vi "CRYGraph Property Window Octave.vi"(9 "TabName":string, 10 "Graph VI Ref":refnum<vi>) -> ()   [LabVIEW 2013]
uses:
  <vilib>/Utility/miscctls.llb/LVRowAndColumnTypeDef.ctl
panel:
  in  "SetFormat":bool
  in  "No Data":bool
  out "CursorLineStyle":string
  out "CursorLineWidth":string
  out "CursorPointStyle":string
  out "CursorStyle":string
  out "Scale Style":u8=5
  out "Interpolation":string
  out "PointStyle":string
  out "LineWidth":string
  out "LineStyle":string
  in  "Property Tab":T1(tab)
  in  "Background Color":u32(colorbox) caption="背景颜色"
  in  "Title Name":string caption="标题名字"
  in  "FormatAxis":u16(ring) items=["X-Axis", "Y-Axis"]
  in  "Notation":i32(listbox)
  in  "PrecisionType":u16(ring) items=["精度位数", "有效数字"]
  in  "PrecisionDigits":u16
  in  "Hide trailing zeros":bool caption="隐藏尾随零"
  in  "Exponent in multiples of 3":bool caption="指数"
  in  "Use minimum field width":bool caption="使用最小场宽度"
  in  "Field Width":u16
  in  "PadType":u16(ring) items=["在左加空格", "在右加空格", "在左加零"]
  in  "Ignore timestamp information":bool caption="忽略时间戳信息"
  in  "TimeFormat":u16(ring) items=["Custom time format", "System time format", "Time unused"]
  in  "Digits":u16 caption="a"
  in  "DateFormat":u16(ring) items=["Custom date format", "System date format", "Date unused"]
  in  "YMD":u16(slide)
  in  "YearShow":u16(slide)
  in  "AMFM":u16(slide)=1
  in  "HMS":u16(slide)=1
  in  "Point/Fill":u32(colorbox) caption="点/填充"
  in  "Fill to":i16(ring) caption="填写" items=["无"=-1, "零"=-2, "-无穷"=-3, "+无穷"=-4]
  in  "Items":u16(ring)
  out "Colors":bool caption="颜色"
  in  "Line":u32(colorbox) caption="线"
  in  "LineStyle4":bool
  in  "LineStyle3":bool
  in  "LineStyle2":bool
  in  "LineStyle0":bool
  in  "LineStyle1":bool
  in  "LineWidth5":bool
  in  "LineWidth1":bool
  in  "LineWidth4":bool
  in  "LineWidth3":bool
  in  "LineWidth2":bool
  in  "LineWidth0":bool
  in  "PointStyle16":bool
  in  "PointStyle15":bool
  in  "PointStyle14":bool
  in  "PointStyle13":bool
  in  "PointStyle12":bool
  in  "PointStyle11":bool
  in  "PointStyle10":bool
  in  "PointStyle9":bool
  in  "PointStyle8":bool
  in  "PointStyle7":bool
  in  "PointStyle6":bool
  in  "PointStyle5":bool
  in  "PointStyle4":bool
  in  "PointStyle3":bool
  in  "PointStyle2":bool
  in  "PointStyle1":bool
  in  "PointStyle0":bool
  in  "Interpolation4":bool
  in  "Interpolation5":bool
  in  "Interpolation3":bool
  in  "Interpolation2":bool
  in  "Interpolation1":bool
  in  "Interpolation0":bool
  in  "Show Plot":bool caption="显示绘图"
  in  "GridStyle":u16(ring)=4
  in  "Minor grid":u32(colorbox) caption="辅网格"
  in  "Major grid":u32(colorbox) caption="主网格"
  in  "Marker text":u32(colorbox) caption="标记文本"
  in  "Minor tick":u32(colorbox) caption="辅刻度"
  in  "Log":bool caption="对数"
  in  "Show scale":bool caption="显示缩放"
  in  "Show scale label":bool caption="显示缩放标签"
  in  "Maximum":dbl caption="最大值"
  in  "Minimum":dbl caption="最小值"
  in  "Autoscale":bool caption="自动缩放"
  in  "Axis Name":string caption="名字"
  in  "Axis":u16(ring)
  in  "Major tick":u32(colorbox) caption="主刻度"
  out "Grid Colors":bool caption="网格颜色"
  out "Scale Style and Colors":bool caption="缩放样式和颜色"
  in  "Show Cursors":bool caption="显示游标"
  in  "Cursor Tab":enum32{"Page 1"}(tab)
  in  "CursorPointStyle16":bool
  in  "CursorPointStyle15":bool
  in  "CursorPointStyle14":bool
  in  "CursorPointStyle13":bool
  in  "CursorPointStyle12":bool
  in  "CursorPointStyle11":bool
  in  "CursorPointStyle10":bool
  in  "CursorPointStyle9":bool
  in  "CursorPointStyle8":bool
  in  "CursorPointStyle7":bool
  in  "CursorPointStyle6":bool
  in  "CursorPointStyle5":bool
  in  "CursorPointStyle4":bool
  in  "CursorPointStyle3":bool
  in  "CursorPointStyle2":bool
  in  "CursorPointStyle1":bool
  in  "CursorPointStyle0":bool
  in  "CursorLineWidth5":bool
  in  "CursorLineWidth1":bool
  in  "CursorLineWidth4":bool
  in  "CursorLineWidth3":bool
  in  "CursorLineWidth2":bool
  in  "CursorLineWidth0":bool
  in  "CursorLineStyle4":bool
  in  "CursorLineStyle3":bool
  in  "CursorLineStyle2":bool
  in  "CursorLineStyle0":bool
  in  "CursorLineStyle1":bool
  in  "Cursor Items":u16(ring)
  in  "CursorStyle8":bool
  in  "CursorStyle4":bool
  in  "CursorStyle5":bool
  in  "CursorStyle7":bool
  in  "CursorStyle6":bool
  in  "CursorStyle3":bool
  in  "CursorStyle2":bool
  in  "CursorStyle1":bool
  in  "CursorStyle0":bool
  in  "Cursor color":u32(colorbox) caption="游标颜色"
  in  "Linked to plot:":u16(ring) caption="连接到游标"
  in  "Link Cursors":bool
  in  "OK":bool
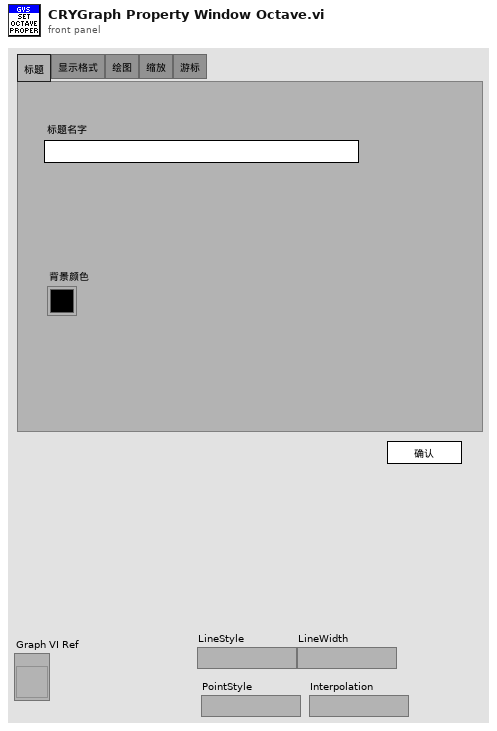
[diagram p1: front panel]
types:
  T1 = enum32{"Title", "Format and Precision", "Plot", "Scale", "Cursor"}
  T2 = enum32{"Page Enabled", "Page Disabled", "Page Disabled & Grayed"}
  T3 = enum8{"Enabled", "Disabled", "Disabled and Grayed Out"}
  T4 = typedef "LVRowAndColumnTypeDef.ctl" = cluster{"Row":i32, "Column":i32}
  T5 = typedef "CRYData Cluster.ctl" = cluster{"Name":string, "Curve":cluster{"x":dbl, "y":dbl, "z":dbl}[], "X data":u16, "Y data":u16, "Z data":u16, "X axis":u16, "Y axis":u16, "Z axis":u16, "X unit":string, "Y unit":string, "Z unit":string, "X dB ref":dbl, "Y dB ref":dbl, "Z dB ref":dbl, "single val":bool, "protected":bool, "display X":bool, "display Y":bool, "display Z":bool, "Test Info":string, "Step No.":i32, "Plot Settings":cluster{"Color":u32, "Interpolation":u8, "Point Style":u8, "Line Style":u8, "Point Color":u32, "Line Width":u8, "Bar Plot Style":u8, "Fill To":i16}, "AutoProtect":bool}
  T6 = cluster{"Notation":i32, "PrecisionType":u16, "PrecisionDigits":u16, "Hide trailing zeros":bool, "Exponent in multiples of 3":bool, "Field Width":u16, "PadType":u16, "Use minimum field width":bool, "TimeFormat":u16, "AMFM":u16, "HMS":u16, "Digits":u16, "DateFormat":u16, "YMD":u16, "YearShow":u16}
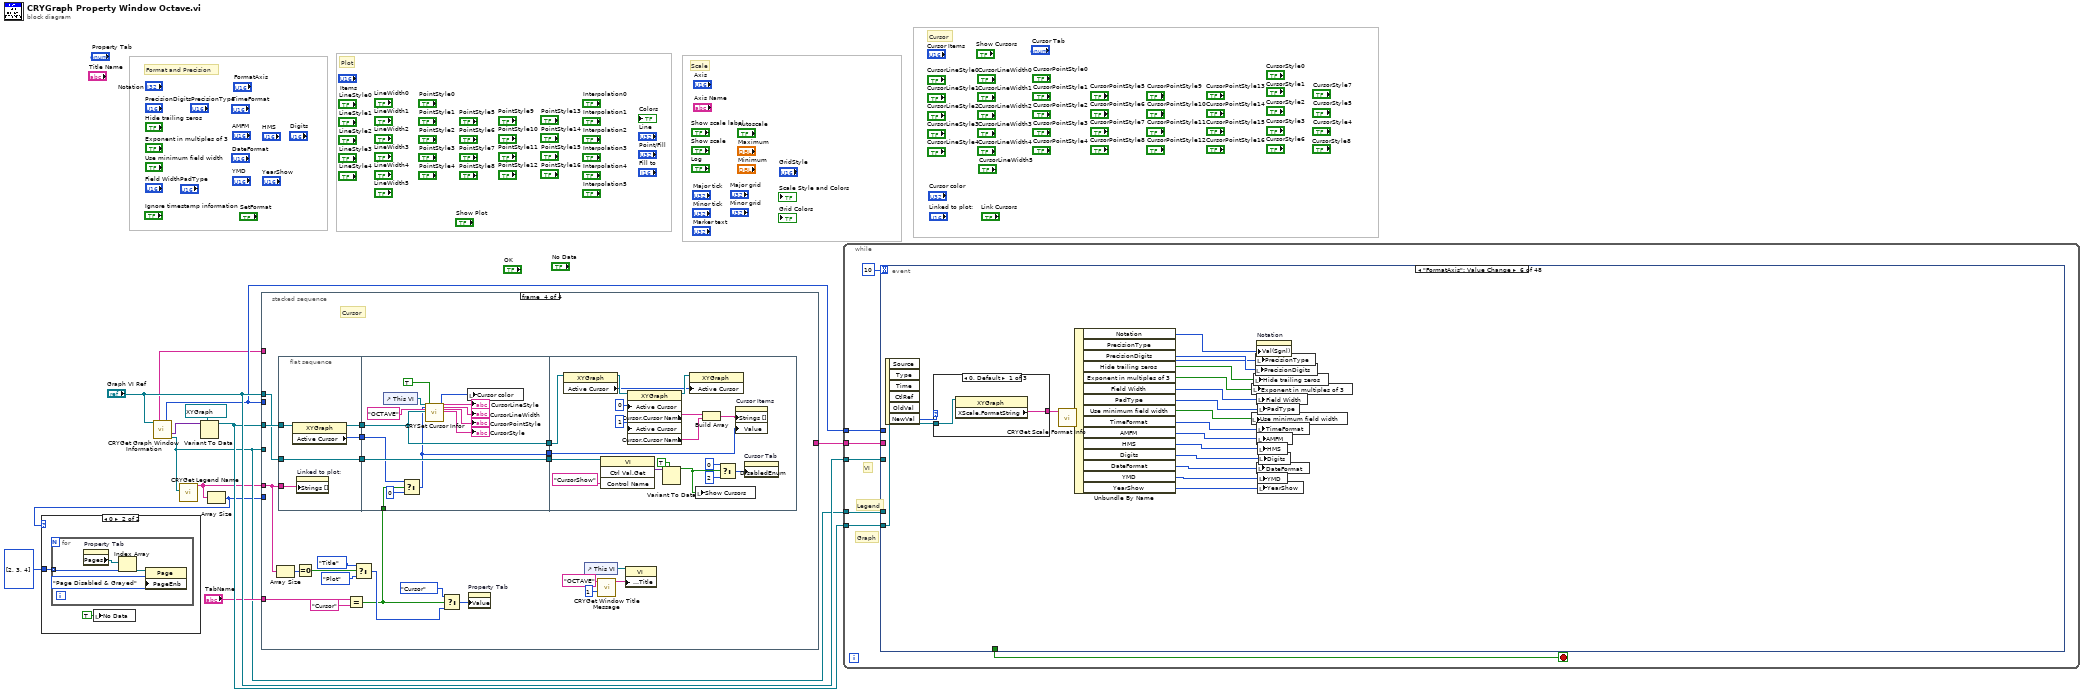
[diagram p0: block diagram]
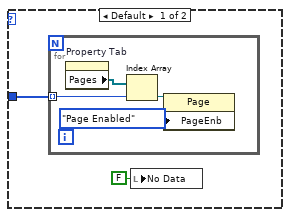
[diagram p2: hidden frame]
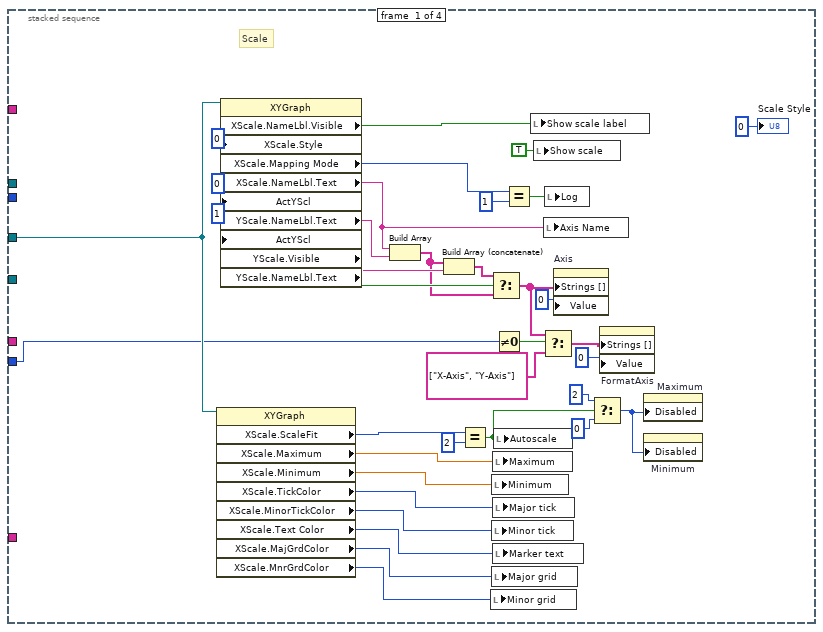
[diagram p3: hidden frame]
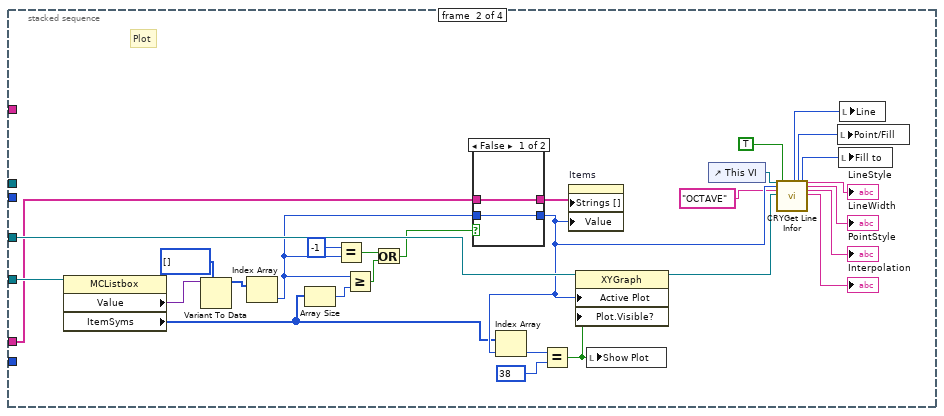
[diagram p4: hidden frame]
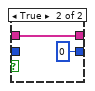
[diagram p5: hidden frame]
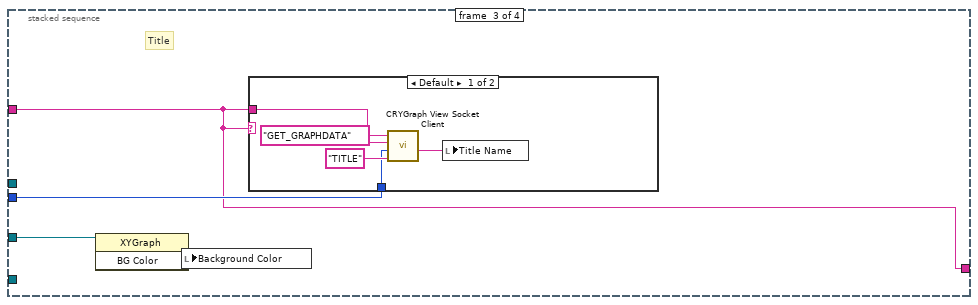
[diagram p6: hidden frame]
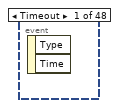
[diagram p8: hidden frame]
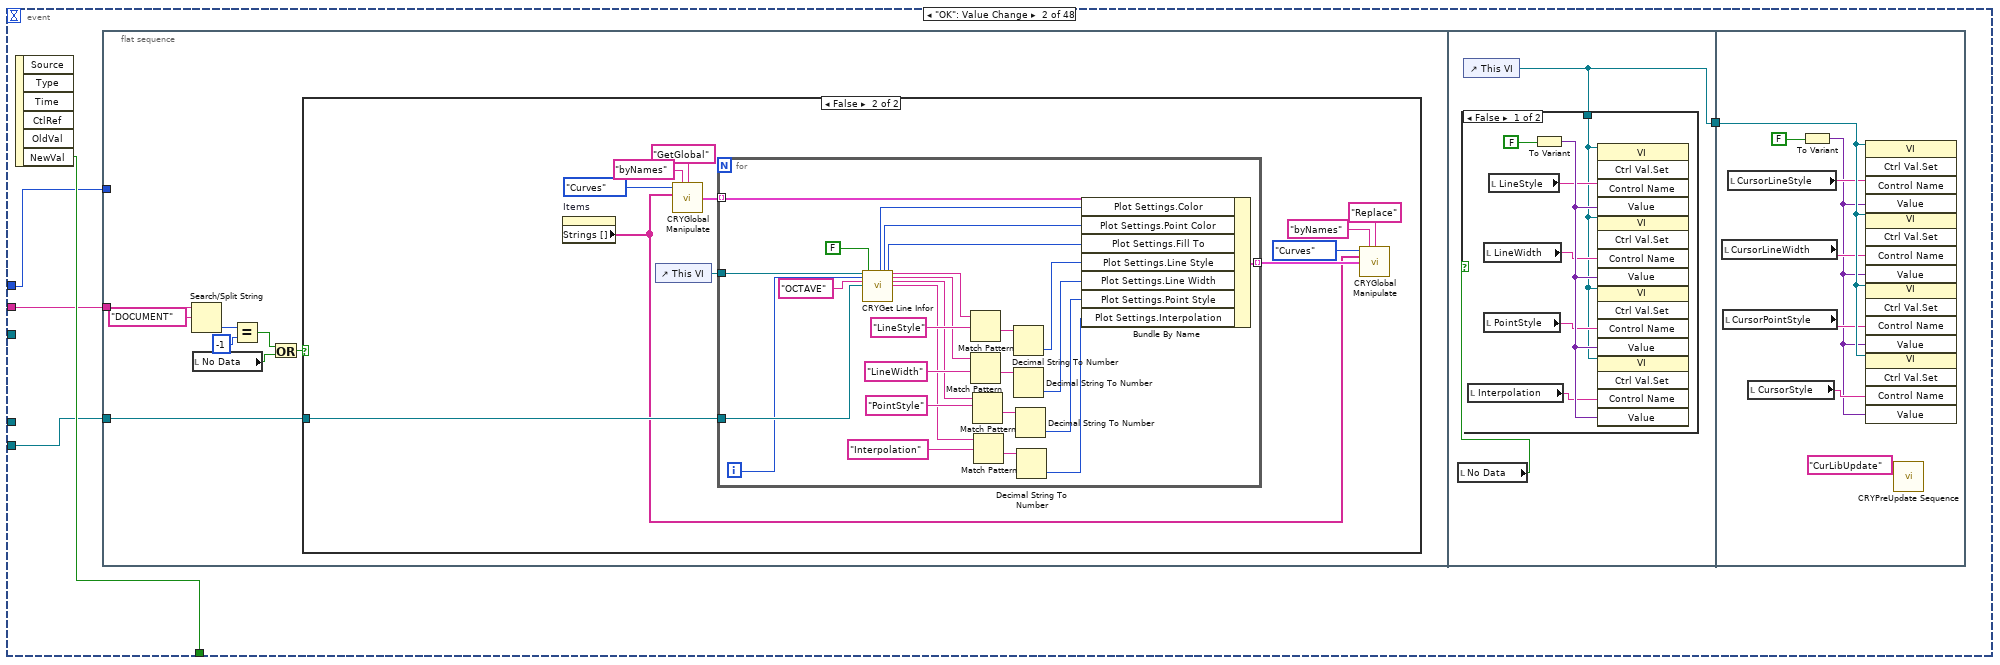
[diagram p9: hidden frame]
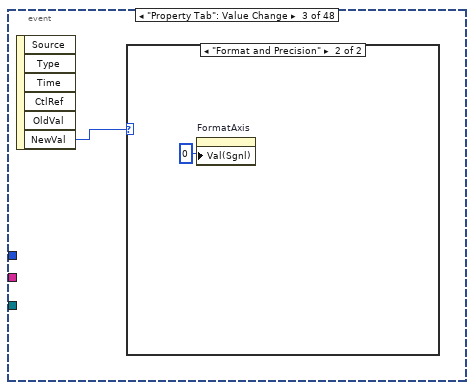
[diagram p12: hidden frame]
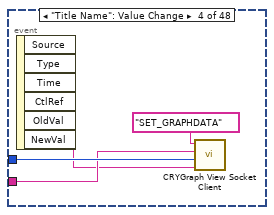
[diagram p14: hidden frame]
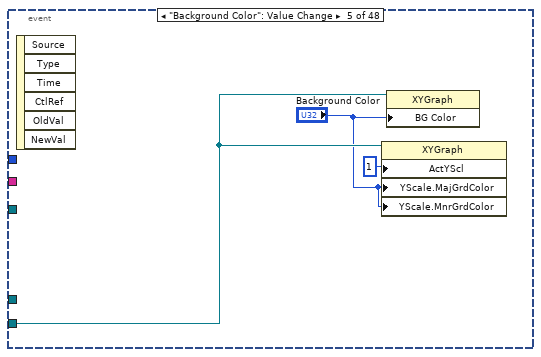
[diagram p15: hidden frame]
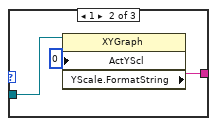
[diagram p16: hidden frame]
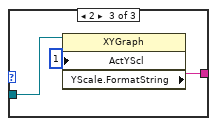
[diagram p17: hidden frame]
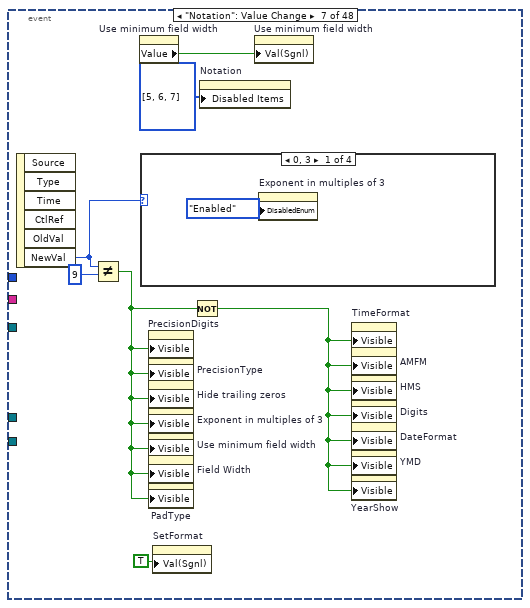
[diagram p18: hidden frame]
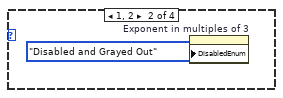
[diagram p19: hidden frame]
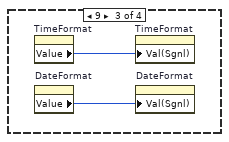
[diagram p20: hidden frame]
diagram:
  # "Format and Precision"
  # "Cursor"
  # "Scale"
  # "Plot"
  n1 = call "CRYGet Graph Window Information.vi"("pGraph VI In"="Graph VI Ref") -> ("Queue Name Out"=w9:string, "Graph Number Out"=w10:i32, "Graph Control Ref Out"=w2:variant, "Legend Ref Out"=w6:refnum<vi>)  [unwired: 2 in, 9 out]
  n2 = call "CRYGet Legend Name.vi"("MCListbox Refnum"=w6) -> ("Names Out"=w5:string[])  [unwired: 1 in, 9 out]
  n3 = Variant To Data(type=refnum<vi> refnum ("XY Graph"), Variant=w2) -> (data=w11:refnum<vi>)  [unwired: 1 in, 1 out]
  n4 = Array Size(array=w5) -> (size(s)=w4:i32)
  n5 = case shown="0" w4 {
    tunnel: i32[] [2, 3, 4] -> [w13 w19]
    frame Default {
      n6 = for {
        tunnel: w13 -> [w16] mode=indexing
        n7 = property on="Property Tab" class="TabCtl (strict)"() -> ("Pages"=w15:refnum<vi>[])  [unwired: 2 in, 2 out]
        n8 = Index Array(array=w15, index=w16) -> (element=w17:refnum<vi>)
        n9 = property class="Page"(reference=w17, "PageEnb"=T2."Page Enabled" ("Page Enabled State")) -> ()  [unwired: 1 in, 2 out]
      }
      n10 = local write "No Data"(FALSE ("No Data")) -> ()
    }
    frame 0 {
      n11 = for {
        tunnel: w19 -> [w21] mode=indexing
        n12 = property on="Property Tab" class="TabCtl (strict)"() -> ("Pages"=w22:refnum<vi>[])  [unwired: 2 in, 2 out]
        n13 = Index Array(array=w22, index=w21) -> (element=w23:refnum<vi>)
        n14 = property class="Page"(reference=w23, "PageEnb"=T2."Page Disabled & Grayed" ("Page Enabled State")) -> ()  [unwired: 1 in, 2 out]
      }
      n15 = local write "No Data"(TRUE ("No Data")) -> ()
    }
  }
  n16 = stacked-sequence {
    tunnel: w11 -> [w60 w88 w97 w125]
    tunnel: "Graph VI Ref" -> [_ _ _ w122]
    tunnel: w6 -> [_ w89 _ _]
    tunnel: w10 -> [_ _ w95 _]
    tunnel: w9 -> [_ _ w94 _]
    tunnel: [_ _ w94 _] -> w8
    tunnel: "TabName" -> [_ _ _ w120]
    tunnel: w5 -> [_ w87 _ w114]
    tunnel: w4 -> [w29 _ _ _]
    frame #0 {
      # "Scale"
      n17 = property class="XYGraph"(reference=w60) -> ("XScale.ScaleFit"=w47:u8, "XScale.Maximum"=w46:dbl, "XScale.Minimum"=w45:dbl, "XScale.TickColor"=w44:u32, "XScale.MinorTickColor"=w43:u32, "XScale.Text Color"=w42:u32, "XScale.MajGrdColor"=w41:u32, "XScale.MnrGrdColor"=w40:u32)  [unwired: 1 in, 2 out]
      n18 = property class="XYGraph"(reference=w60, "XScale.Style"=u8 0 ("X Scale.Style"), "ActYScl"=0 ("Active Y Scale"), "ActYScl"=1 ("Active Y Scale")) -> ("XScale.NameLbl.Visible"=w58:bool, "XScale.Mapping Mode"=w56:u8, "XScale.NameLbl.Text"=w53:string, "YScale.NameLbl.Text"=w51:string, "YScale.Visible"=w34:bool, "YScale.NameLbl.Text"=w33:string)  [unwired: 1 in, 2 out]
      n19 = Build Array(w53, w51) -> (w31:string[])
      n20 = Build Array (concatenate)(w31, w33) -> (w32:string[])
      n21 = Equal?(x=w47, y=u8 2 ("X Scale.Scale Fit")) -> (x = y?=w36:bool)
      n22 = Select(t=w32, s=w34, f=w31) -> (s? t:f=w27:string[])
      n23 = local write "Minor grid"(w40) -> ()
      n24 = local write "Minimum"(w45) -> ()
      n25 = local write "Minor tick"(w43) -> ()
      n26 = local write "Major grid"(w41) -> ()
      n27 = local write "Maximum"(w46) -> ()
      n28 = local write "Major tick"(w44) -> ()
      n29 = local write "Marker text"(w42) -> ()
      n30 = Not Equal To 0?(x=w29) -> (x != 0?=w28:bool)
      n31 = local write "Autoscale"(w36) -> ()
      n32 = Equal?(x=w56, y=u8 1) -> (x = y?=w57:bool)
      n33 = local write "Show scale label"(w58) -> ()
      n34 = local write "Show scale"(TRUE ("Show scale")) -> ()
      n35 = Select(t=w27, s=w28, f=string[] ["X-Axis", "Y-Axis"]) -> (s? t:f=w25:string[])
      n36 = local write "Axis Name"(w53) -> ()
      n37 = local write "Log"(w57) -> ()
      n38 = property on="Axis" class="Ring (strict)"("Strings []"=w27, "Value"=0) -> ()  [unwired: 2 in, 2 out]
      n39 = Select(t=u8 2 ("X Scale.Scale Fit"), s=w36, f=u8 0 ("X Scale.Scale Fit")) -> (s? t:f=w37:u8)
      n40 = property on="FormatAxis" class="Ring (strict)"("Strings []"=w25, "Value"=0) -> ()  [unwired: 2 in, 2 out]
      n41 = property on="Maximum" class="DigNum (strict)"("Disabled"=w37) -> ()  [unwired: 2 in, 2 out]
      n42 = property on="Minimum" class="DigNum (strict)"("Disabled"=w37) -> ()  [unwired: 2 in, 2 out]
      "Scale Style" <- u8 0 ("X Scale.Scale Fit")
    }
    frame #1 {
      # "Plot"
      n43 = property class="MCListbox"(reference=w89) -> ("Value"=w81:variant, "ItemSyms"=w63:i32[])  [unwired: 1 in, 2 out]
      n44 = Variant To Data(type=i32[] [], Variant=w81) -> (data=w68:i32[])  [unwired: 1 in, 1 out]
      n45 = Index Array(array=w68) -> (element=w61:i32)  [unwired: 1 in]
      n46 = Array Size(array=w63) -> (size(s)=w66:i32)
      n47 = Equal?(x=-1, y=w61) -> (x = y?=w65:bool)
      n48 = Greater Or Equal?(x=w61, y=w66) -> (x >= y?=w64:bool)
      n49 = Or(x=w65, y=w64) -> (x .or. y?=w62:bool)
      n50 = case shown="False" w62 {
        tunnel: w87 -> [w91 w93]
        tunnel: [w91 w93] -> w86
        tunnel: [w90 0 ("Value")] -> w80
        tunnel: w61 -> [w90 _]
        frame False {
        }
        frame True {
        }
      }
      n51 = Index Array(array=w63, index=w80) -> (element=w83:i32)
      n52 = Equal?(x=w83, y=38) -> (x = y?=w82:bool)
      n53 = property on="Items" class="Ring (strict)"("Strings []"=w86, "Value"=w80) -> ()  [unwired: 2 in, 2 out]
      n54 = property class="XYGraph"(reference=w88, "Active Plot"=w80, "Plot.Visible?"=w82) -> (reference out=w85:refnum<vi>)  [unwired: 1 in, 1 out]
      n55 = local write "Show Plot"(w82) -> ()
      n56 = control-ref of="This VI"() -> (w79:refnum<vi>)
      n57 = call "CRYGet Line Infor.vi"("This VI"=w79, "Active Plot Number"=w80, "Graph Type"="OCTAVE", "XY Graph Control Ref"=w85, "Property Set?"=TRUE) -> ("Line"=w72:u32, "Point/Fill"=w70:u32, "Fill to"=w71:i16, "LineStyle"=→"LineStyle":string, "LineWidth"=→"LineWidth":string, "PointStyle"=→"PointStyle":string, "Interpolation"=→"Interpolation":string)  [unwired: 16 in]
      n58 = local write "Point/Fill"(w70) -> ()
      n59 = local write "Fill to"(w71) -> ()
      n60 = local write "Line"(w72) -> ()
    }
    frame #2 {
      # "Title"
      n61 = property class="XYGraph"(reference=w97) -> ("BG Color"=w96:u32)  [unwired: 1 in, 2 out]
      n62 = local write "Background Color"(w96) -> ()
      n63 = case shown="Default" w94 {
        tunnel: w95 -> [w100 _]
        tunnel: w94 -> [w99 _]
        frame Default {
          n64 = call "CRYGraph View Socket Client.vi"("sOption"="TITLE", "nData"=w100, "sData"=w99, "sAction"="GET_GRAPHDATA") -> ("sData Out"=w98:string)  [unwired: 4 in, 3 out]
          n65 = local write "Title Name"(w98) -> ()
        }
        frame "test DataView" {
        }
      }
    }
    frame #3 {
      # "Cursor"
      n66 = Array Size(array=w114) -> (size(s)=w121:i32)
      n67 = flat-sequence {
        tunnel: w122 -> [w130]
        tunnel: w125 -> [w128]
        tunnel: [w127] -> w116
        tunnel: [w130] -> w115
        tunnel: w114 -> [w129]
        tunnel: [w126] -> w112
        tunnel: [w144] -> w124
        tunnel: [w135] -> w123
        tunnel: w116 -> [w144]
        tunnel: w115 -> [w135]
        tunnel: w113 -> [w133]
        tunnel: w112 -> [w132]
        tunnel: [w131] -> w111
        tunnel: w124 -> [w148]
        tunnel: w123 -> [w154]
        tunnel: w111 -> [w145]
        frame #0 {
          n68 = property class="XYGraph"(reference=w128) -> (reference out=w127:refnum<vi>, "Active Cursor"=w126:u32)  [unwired: 1 in, 1 out]
          n69 = property on="Linked to plot:" class="Ring (strict)"("Strings []"=w129) -> ()  [unwired: 2 in, 2 out]
        }
        frame #1 {
          n70 = control-ref of="This VI"() -> (w143:refnum<vi>)
          n71 = Select(t=w132, s=w133, f=u32 0 ("Active Cursor")) -> (s? t:f=w131:u32)
          n72 = call "CRYSet Cursor Infor.vi"("This VI"=w143, "Active Cursor"=w131, "Graph Type"="OCTAVE", "XY Graph Ref"=w144, "Property Set?"=TRUE) -> ("Cursor Color"=w136:u32, "CursorLineStyle"=→"CursorLineStyle":string, "CursorLineWidth"=→"CursorLineWidth":string, "CursorPointStyle"=→"CursorPointStyle":string, "CursorStyle"=→"CursorStyle":string)  [unwired: 17 in, 1 out]
          n73 = local write "Cursor color"(w136) -> ()
        }
        frame #2 {
          n74 = property class="XYGraph"(reference=w148) -> (reference out=w147:refnum<vi>, "Active Cursor"=w146:u32)  [unwired: 1 in, 1 out]
          n75 = invoke class="VI" method="Ctrl Val.Get"(reference=w154, "Control Name"="CursorShow") -> ("Get Control Value Variant"=w152:variant)  [unwired: 2 in, 3 out]
          n76 = property class="XYGraph"(reference=w147, "Active Cursor"=u32 0, "Active Cursor"=u32 1) -> (reference out=w149:refnum<vi>, "Cursor.Cursor Name"=w157:string, "Cursor.Cursor Name"=w158:string)  [unwired: 1 in, 1 out]
          n77 = Variant To Data(type=TRUE ("Visible"), Variant=w152) -> (data=w150:bool)  [unwired: 1 in, 1 out]
          n78 = property class="XYGraph"(reference=w149, "Active Cursor"=w146) -> ()  [unwired: 1 in, 2 out]
          n79 = local write "Show Cursors"(w150) -> ()
          n80 = Build Array(w157, w158) -> (w159:string[])
          n81 = Select(t=0, s=w150, f=2) -> (s? t:f=w160:i32)
          n82 = property on="Cursor Items" class="Ring (strict)"("Strings []"=w159, "Value"=w145) -> ()  [unwired: 2 in, 2 out]
          n83 = property on="Cursor Tab" class="TabCtl (strict)"("DisabledEnum"=w160) -> ()  [unwired: 2 in, 2 out]
        }
      }
      n84 = Equal To 0?(x=w121) -> (x = 0?=w118:bool)
      n85 = Equal?(x=w120, y="Cursor" ("Graph Type")) -> (x = y?=w113:bool)
      n86 = Select(t=T1."Title" ("Tab Control"), s=w118, f=T1."Plot" ("Tab Control")) -> (s? t:f=w117:T1)
      n87 = Select(t=T1."Cursor" ("Tab Control"), s=w113, f=w117) -> (s? t:f=w110:T1)
      n88 = property on="Property Tab" class="TabCtl (strict)"("Value"=w110) -> ()  [unwired: 2 in, 2 out]
      n89 = control-ref of="This VI"() -> (w103:refnum<vi>)
      n90 = call "CRYGet Window Title Message.vi"("No"=1 ("Error No"), "Kind"="OCTAVE") -> ("Multibyte String"=w104:string)  [unwired: 4 in, 5 out]
      n91 = property class="VI"(reference=w103, "Front Panel.Title"=w104) -> ()  [unwired: 1 in, 2 out]
    }
  }
  n92 = while {
    tunnel: w11 -> [w168]
    tunnel: "Graph VI Ref" -> [w167]
    tunnel: w6 -> [w165]
    tunnel: w8 -> [w164]
    tunnel: w10 -> [w163]
    stop <- w169 stop-if-true
    # "VI"
    # "Legend"
    # "Graph"
    n93 = event shown="[5] \"FormatAxis\": Value Change" {
      selector: _ -> [_ _ _ _ _ _ _ _ _ _ _ _ _ _ _ _ _ _ _ _ _ _ _ _ _ _ _ _ _ _ _ _ _ _ _ _ _ _ _ _ _ _ _ _ _ _ _ _]
      dyn-events: _ -> [_ _ _ _ _ _ _ _ _ _ _ _ _ _ _ _ _ _ _ _ _ _ _ _ _ _ _ _ _ _ _ _ _ _ _ _ _ _ _ _ _ _ _ _ _ _ _ _]
      timeout: 10 -> [_ _ _ _ _ _ _ _ _ _ _ _ _ _ _ _ _ _ _ _ _ _ _ _ _ _ _ _ _ _ _ _ _ _ _ _ _ _ _ _ _ _ _ _ _ _ _ _]
      tunnel: [_ w174 _ _ _ _ _ _ _ _ _ _ _ _ _ _ _ _ _ _ _ _ _ _ _ _ _ _ _ _ _ _ _ _ _ _ _ _ _ _ _ _ _ _ _ _ _ _] -> w169
      tunnel: w168 -> [_ w173 _ _ w244 w255 _ _ _ _ _ _ _ _ _ w330 w476 w508 w540 w572 w602 w639 w649 w659 w676 w698 w742 w754 w769 w781 w795 w807 w818 w829 w839 w851 w869 w906 w917 _ w934 w954 w975 w996 w1017 w1042 w1051 _]
      tunnel: w167 -> [_ _ _ _ _ _ _ _ _ _ _ _ _ _ _ _ _ _ _ _ _ _ _ _ _ _ _ _ _ _ _ _ _ _ _ _ w863 _ _ w930 _ _ _ _ _ w1043 _ _]
      tunnel: w165 -> [_ _ _ _ _ _ _ _ _ _ _ _ _ _ _ _ w475 w507 w539 w571 w604 w638 w645 w657 w673 _ _ _ _ _ _ _ _ _ _ _ _ _ _ _ _ _ _ _ _ _ _ _]
      tunnel: w164 -> [_ w171 _ w240 _ _ _ _ _ _ _ _ _ _ _ _ w474 w506 w538 w570 _ w632 w647 w656 _ _ _ _ _ _ _ _ _ _ _ _ _ _ _ _ _ _ _ _ _ _ _ _]
      tunnel: w163 -> [_ w170 _ w241 _ _ _ _ _ _ _ _ _ _ _ _ _ _ _ _ _ _ _ _ _ _ _ _ _ _ _ _ _ _ _ _ _ _ _ _ _ _ _ _ _ _ _ _]
      event Timeout {
        n94 = event-data() -> ()  [unwired: 3 out]
      }
      event "OK": Value Change {
        n95 = event-data() -> ("NewVal"=w174:bool)  [unwired: 6 out]
        n96 = flat-sequence {
          tunnel: w173 -> [w175]
          tunnel: w171 -> [w177]
          tunnel: w170 -> [_]
          tunnel: [w221] -> w172
          tunnel: w172 -> [w236]
          frame #0 {
            n97 = Search/Split String(string=w177, search string/char (-)="DOCUMENT" ("regular expression")) -> (offset of match=w181:i32)  [unwired: 1 in, 2 out]
            n98 = local read "No Data"() -> (w178:bool)
            n99 = Equal?(x=w181, y=-1) -> (x = y?=w179:bool)
            n100 = Or(x=w179, y=w178) -> (x .or. y?=w176:bool)
            n101 = case shown="False" w176 {
              tunnel: w175 -> [_ w192]
              frame True {
              }
              frame False {
                n102 = property on="Items" class="Ring (strict)"() -> ("Strings []"=w184:string[])  [unwired: 2 in, 2 out]
                n103 = control-ref of="This VI"() -> (w193:refnum<vi>)
                n104 = call "CRYGlobal Manipulate.vi"("Type"=enum16{"Curves", "Values", "Results", "WFM"}."Curves", "sOption"="byNames", "sAction"="GetGlobal", "sData"=w184) -> ("Curves Out"=w188:T5[])  [unwired: 5 in, 6 out]
                n105 = for {
                  tunnel: w193 -> [w218]
                  tunnel: w192 -> [w217]
                  tunnel: w188 -> [w195] mode=indexing
                  tunnel: [w194] -> w187 mode=indexing
                  i -> [w201]
                  n106 = call "CRYGet Line Infor.vi"("This VI"=w218, "Active Plot Number"=w201, "Graph Type"="OCTAVE", "XY Graph Control Ref"=w217, "Property Set?"=FALSE) -> ("Line"=w196:u32, "Point/Fill"=w197:u32, "Fill to"=w198:i16, "LineStyle"=w208:string, "LineWidth"=w204:string, "PointStyle"=w203:string, "Interpolation"=w202:string)  [unwired: 16 in]
                  n107 = Match Pattern(string=w208, regular expression="LineStyle") -> (after substring=w214:string)  [unwired: 4 out]
                  n108 = Match Pattern(string=w204, regular expression="LineWidth") -> (after substring=w215:string)  [unwired: 4 out]
                  n109 = Match Pattern(string=w203, regular expression="PointStyle") -> (after substring=w213:string)  [unwired: 4 out]
                  n110 = Match Pattern(string=w202, regular expression="Interpolation") -> (after substring=w210:string)  [unwired: 4 out]
                  n111 = Decimal String To Number(string=w214) -> (number=w207:i32)  [unwired: 3 out]
                  n112 = Decimal String To Number(string=w215) -> (number=w206:i32)  [unwired: 3 out]
                  n113 = Decimal String To Number(string=w213) -> (number=w205:i32)  [unwired: 3 out]
                  n114 = Decimal String To Number(string=w210) -> (number=w200:i32)  [unwired: 3 out]
                  n115 = Bundle By Name(cluster=w195, "Plot Settings.Color"=w196, "Plot Settings.Point Color"=w197, "Plot Settings.Fill To"=w198, "Plot Settings.Line Style"=w207, "Plot Settings.Line Width"=w206, "Plot Settings.Point Style"=w205, "Plot Settings.Interpolation"=w200) -> (w194:T5)
                }
                n116 = call "CRYGlobal Manipulate.vi"("Type"=enum16{"Curves", "Values", "Results", "WFM"}."Curves", "sOption"="byNames", "sAction"="Replace", "sData"=w184, "Curves"=w187) -> ()  [unwired: 4 in, 7 out]
              }
            }
          }
          frame #1 {
            n117 = local read "No Data"() -> (w220:bool)
            n118 = control-ref of="This VI"() -> (w221:refnum<vi>)
            n119 = case shown="False" w220 {
              tunnel: w221 -> [w222 _]
              frame False {
                n120 = local read "Interpolation"() -> (w223:string)
                n121 = local read "LineWidth"() -> (w225:string)
                n122 = local read "PointStyle"() -> (w224:string)
                n123 = local read "LineStyle"() -> (w226:string)
                n124 = To Variant(anything=FALSE) -> (Variant=w228:variant)
                n125 = invoke class="VI" method="Ctrl Val.Set"(reference=w222, "Control Name"=w226, "Value"=w228) -> ()  [unwired: 2 in, 5 out]
                n126 = invoke class="VI" method="Ctrl Val.Set"(reference=w222, "Control Name"=w225, "Value"=w228) -> ()  [unwired: 2 in, 5 out]
                n127 = invoke class="VI" method="Ctrl Val.Set"(reference=w222, "Control Name"=w224, "Value"=w228) -> ()  [unwired: 2 in, 5 out]
                n128 = invoke class="VI" method="Ctrl Val.Set"(reference=w222, "Control Name"=w223, "Value"=w228) -> ()  [unwired: 2 in, 5 out]
              }
              frame True {
              }
            }
          }
          frame #2 {
            n129 = local read "CursorLineWidth"() -> (w233:string)
            n130 = local read "CursorPointStyle"() -> (w234:string)
            n131 = local read "CursorLineStyle"() -> (w232:string)
            n132 = local read "CursorStyle"() -> (w235:string)
            n133 = To Variant(anything=FALSE) -> (Variant=w230:variant)
            n134 = invoke class="VI" method="Ctrl Val.Set"(reference=w236, "Control Name"=w232, "Value"=w230) -> ()  [unwired: 2 in, 5 out]
            n135 = invoke class="VI" method="Ctrl Val.Set"(reference=w236, "Control Name"=w233, "Value"=w230) -> ()  [unwired: 2 in, 5 out]
            n136 = invoke class="VI" method="Ctrl Val.Set"(reference=w236, "Control Name"=w234, "Value"=w230) -> ()  [unwired: 2 in, 5 out]
            n137 = invoke class="VI" method="Ctrl Val.Set"(reference=w236, "Control Name"=w235, "Value"=w230) -> ()  [unwired: 2 in, 5 out]
            n138 = call "CRYPreUpdate Sequence.vi"("EventName"="CurLibUpdate") -> ()  [unwired: 15 in]
          }
        }
      }
      event "Property Tab": Value Change {
        n139 = event-data() -> ("NewVal"=w237:T1)  [unwired: 6 out]
        n140 = case shown="\"Format and Precision\"" w237 {
          frame "Title", Default {
          }
          frame "Format and Precision" {
            n141 = property on="FormatAxis" class="Ring (strict)"("Val(Sgnl)"=u16 0 ("Value (Signaling)")) -> ()  [unwired: 2 in, 2 out]
          }
        }
      }
      event "Title Name": Value Change {
        n142 = event-data() -> ("NewVal"=w239:string)  [unwired: 6 out]
        n143 = call "CRYGraph View Socket Client.vi"("sOption"=w239, "nData"=w241, "sData"=w240, "sAction"="SET_GRAPHDATA") -> ()  [unwired: 4 in, 4 out]
      }
      event "Background Color": Value Change {
        n144 = event-data() -> ()  [unwired: 7 out]
        n145 = property on="Property Node" class="XYGraph"(reference=w244, "ActYScl"=1 ("Active Y Scale"), "YScale.MajGrdColor"="Background Color", "YScale.MnrGrdColor"="Background Color") -> ()  [unwired: 1 in, 2 out]
        n146 = property class="XYGraph"(reference=w244, "BG Color"="Background Color") -> ()  [unwired: 1 in, 2 out]
      }
      event "FormatAxis": Value Change {
        n147 = event-data() -> ("NewVal"=w256:u16)  [unwired: 6 out]
        n148 = case shown="0, Default" w256 {
          tunnel: w255 -> [w266 w269 w272]
          tunnel: [w265 w267 w270] -> w263
          frame 0, Default {
            n149 = property class="XYGraph"(reference=w266) -> ("XScale.FormatString"=w265:string)  [unwired: 1 in, 2 out]
          }
          frame 1 {
            n150 = property class="XYGraph"(reference=w269, "ActYScl"=0 ("Active Y Scale")) -> ("YScale.FormatString"=w267:string)  [unwired: 1 in, 2 out]
          }
          frame 2 {
            n151 = property class="XYGraph"(reference=w272, "ActYScl"=1 ("Active Y Scale")) -> ("YScale.FormatString"=w270:string)  [unwired: 1 in, 2 out]
          }
        }
        n152 = call "CRYGet Scale Format Info.vi"("FormatString"=w263) -> ("ScaleFormat"=w264:T6)  [unwired: 10 in]
        n153 = Unbundle By Name(w264) -> ("Notation"=w257:i32, "PrecisionType"=w253:u16, "PrecisionDigits"=w254:u16, "Hide trailing zeros"=w258:bool, "Exponent in multiples of 3"=w259:bool, "Field Width"=w260:u16, "PadType"=w262:u16, "Use minimum field width"=w261:bool, "TimeFormat"=w246:u16, "AMFM"=w247:u16, "HMS"=w248:u16, "Digits"=w249:u16, "DateFormat"=w250:u16, "YMD"=w251:u16, "YearShow"=w252:u16)
        n154 = local write "Use minimum field width"(w261) -> ()
        n155 = local write "Exponent in multiples of 3"(w259) -> ()
        n156 = local write "Hide trailing zeros"(w258) -> ()
        n157 = local write "PrecisionDigits"(w254) -> ()
        n158 = local write "PrecisionType"(w253) -> ()
        n159 = local write "Field Width"(w260) -> ()
        n160 = local write "TimeFormat"(w246) -> ()
        n161 = local write "DateFormat"(w250) -> ()
        n162 = property on="Notation" class="LstBox (strict)"("Val(Sgnl)"=w257) -> ()  [unwired: 2 in, 2 out]
        n163 = local write "AMFM"(w247) -> ()
        n164 = local write "PadType"(w262) -> ()
        n165 = local write "HMS"(w248) -> ()
        n166 = local write "YMD"(w251) -> ()
        n167 = local write "YearShow"(w252) -> ()
        n168 = local write "Digits"(w249) -> ()
      }
      event "Notation": Value Change {
        n169 = event-data() -> ("NewVal"=w274:i32)  [unwired: 6 out]
        n170 = Not Equal?(x=w274, y=9) -> (x != y?=w276:bool)
        n171 = property on="Use minimum field width" class="Bool (strict)"() -> ("Value"=w277:bool)  [unwired: 2 in, 2 out]
        n172 = case shown="0, 3" w274 {
          frame 0, 3 {
            n173 = property on="Exponent in multiples of 3" class="Bool (strict)"("DisabledEnum"=T3."Enabled" ("Disabled")) -> ()  [unwired: 2 in, 2 out]
          }
          frame 1, 2 {
            n174 = property on="Exponent in multiples of 3" class="Bool (strict)"("DisabledEnum"=T3."Disabled and Grayed Out" ("Disabled")) -> ()  [unwired: 2 in, 2 out]
          }
          frame 9 {
            n175 = property on="TimeFormat" class="Ring (strict)"() -> ("Value"=w282:u16)  [unwired: 2 in, 2 out]
            n176 = property on="DateFormat" class="Ring (strict)"() -> ("Value"=w283:u16)  [unwired: 2 in, 2 out]
            n177 = property on="TimeFormat" class="Ring (strict)"("Val(Sgnl)"=w282) -> ()  [unwired: 2 in, 2 out]
            n178 = property on="DateFormat" class="Ring (strict)"("Val(Sgnl)"=w283) -> ()  [unwired: 2 in, 2 out]
          }
          frame Default {
          }
        }
        n179 = property on="PrecisionDigits" class="DigNum (strict)"("Visible"=w276) -> ()  [unwired: 2 in, 2 out]
        n180 = property on="PrecisionType" class="Ring (strict)"("Visible"=w276) -> ()  [unwired: 2 in, 2 out]
        n181 = property on="Hide trailing zeros" class="Bool (strict)"("Visible"=w276) -> ()  [unwired: 2 in, 2 out]
        n182 = property on="Exponent in multiples of 3" class="Bool (strict)"("Visible"=w276) -> ()  [unwired: 2 in, 2 out]
        n183 = property on="Use minimum field width" class="Bool (strict)"("Visible"=w276) -> ()  [unwired: 2 in, 2 out]
        n184 = property on="Field Width" class="DigNum (strict)"("Visible"=w276) -> ()  [unwired: 2 in, 2 out]
        n185 = property on="PadType" class="Ring (strict)"("Visible"=w276) -> ()  [unwired: 2 in, 2 out]
        n186 = property on="SetFormat" class="Bool (strict)"("Val(Sgnl)"=TRUE ("Value (Signaling)")) -> ()  [unwired: 2 in, 2 out]
        n187 = Not(x=w276) -> (.not. x?=w273:bool)
        n188 = property on="Notation" class="LstBox (strict)"("Disabled Items"=i32[] [5, 6, 7]) -> ()  [unwired: 2 in, 2 out]
        n189 = property on="Use minimum field width" class="Bool (strict)"("Val(Sgnl)"=w277) -> ()  [unwired: 2 in, 2 out]
        n190 = property on="TimeFormat" class="Ring (strict)"("Visible"=w273) -> ()  [unwired: 2 in, 2 out]
        n191 = property on="AMFM" class="Slide (strict)"("Visible"=w273) -> ()  [unwired: 2 in, 2 out]
        n192 = property on="HMS" class="Slide (strict)"("Visible"=w273) -> ()  [unwired: 2 in, 2 out]
        n193 = property on="Digits" class="DigNum (strict)"("Visible"=w273) -> ()  [unwired: 2 in, 2 out]
        n194 = property on="DateFormat" class="Ring (strict)"("Visible"=w273) -> ()  [unwired: 2 in, 2 out]
        n195 = property on="YMD" class="Slide (strict)"("Visible"=w273) -> ()  [unwired: 2 in, 2 out]
        n196 = property on="YearShow" class="Slide (strict)"("Visible"=w273) -> ()  [unwired: 2 in, 2 out]
      }
      event "PrecisionType", "PrecisionDigits", "Hide trailing zeros", "Exponent in multiples of 3", "PadType": Value Change {
        n197 = event-data() -> ()  [unwired: 7 out]
        n198 = property on="SetFormat" class="Bool (strict)"("Val(Sgnl)"=TRUE ("Value (Signaling)")) -> ()  [unwired: 2 in, 2 out]
      }
      event "Use minimum field width": Value Change {
        n199 = event-data() -> ("NewVal"=w289:bool)  [unwired: 6 out]
        n200 = property on="Field Width" class="DigNum (strict)"() -> ("Value"=w291:u16)  [unwired: 2 in, 2 out]
        n201 = Equal To 0?(x=w291) -> (x = 0?=w295:bool)
        n202 = Select(t=u16 1 ("Field Width"), s=w295, f=w291) -> (s? t:f=w296:u16)
        n203 = Select(t=T3."Enabled" ("Disabled"), s=w289, f=T3."Disabled and Grayed Out") -> (s? t:f=w285:T3)
        n204 = Select(t=w296, s=w289, f=u16 0 ("Field Width")) -> (s? t:f=w288:u16)
        n205 = property on="Field Width" class="DigNum (strict)"("Value"=w288) -> (error out=w286:errorcluster)  [unwired: 2 in, 1 out]
        n206 = property on="Field Width" class="DigNum (strict)"("DisabledEnum"=w285) -> ()  [unwired: 2 in, 2 out]
        n207 = property on="PadType" class="Ring (strict)"("DisabledEnum"=w285) -> ()  [unwired: 2 in, 2 out]
        n208 = property on="SetFormat" class="Bool (strict)"(error in=w286, "Val(Sgnl)"=TRUE ("Value (Signaling)")) -> ()  [unwired: 1 in, 2 out]
      }
      event "Field Width": Value Change {
        n209 = event-data() -> ("NewVal"=w299:u16)  [unwired: 6 out]
        n210 = property on="SetFormat" class="Bool (strict)"("Val(Sgnl)"=TRUE ("Value (Signaling)")) -> ()  [unwired: 2 in, 2 out]
        n211 = Equal To 0?(x=w299) -> (x = 0?=w302:bool)
        n212 = Select(t=T3."Disabled and Grayed Out" ("Disabled"), s=w302, f=T3."Enabled" ("Disabled")) -> (s? t:f=w298:T3)
        n213 = Select(t=FALSE ("x = 0?"), s=w302, f=TRUE ("x = 0?")) -> (s? t:f=w297:bool)
        n214 = property on="Field Width" class="DigNum (strict)"("DisabledEnum"=w298) -> ()  [unwired: 2 in, 2 out]
        n215 = property on="PadType" class="Ring (strict)"("DisabledEnum"=w298) -> ()  [unwired: 2 in, 2 out]
        n216 = property on="Use minimum field width" class="Bool (strict)"("Value"=w297) -> ()  [unwired: 2 in, 2 out]
      }
      event "TimeFormat": Value Change {
        n217 = event-data() -> ("NewVal"=w309:u16)  [unwired: 6 out]
        n218 = case shown="0, Default" w309 {
          tunnel: [T3."Enabled" ("Disabled") T3."Disabled and Grayed Out" ("Disabled") T3."Disabled and Grayed Out" ("Disabled")] -> w307
          tunnel: [T3."Enabled" ("Disabled") T3."Enabled" ("Disabled") T3."Disabled and Grayed Out" ("Disabled")] -> w306
          frame 0, Default {
            n219 = property on="HMS" class="Slide (strict)"() -> ("Value"=w310:u16)  [unwired: 2 in, 2 out]
            n220 = property on="HMS" class="Slide (strict)"("Val(Sgnl)"=w310) -> ()  [unwired: 2 in, 2 out]
          }
          frame 1 {
          }
          frame 2 {
          }
        }
        n221 = property on="SetFormat" class="Bool (strict)"("Val(Sgnl)"=TRUE ("Value (Signaling)")) -> ()  [unwired: 2 in, 2 out]
        n222 = property on="Digits" class="DigNum (strict)"("DisabledEnum"=w306) -> ()  [unwired: 2 in, 2 out]
        n223 = property on="HMS" class="Slide (strict)"("DisabledEnum"=w307) -> ()  [unwired: 2 in, 2 out]
        n224 = property on="AMFM" class="Slide (strict)"("DisabledEnum"=w307) -> ()  [unwired: 2 in, 2 out]
      }
      event "AMFM", "Digits", "YMD", "YearShow": Value Change {
        n225 = event-data() -> ()  [unwired: 7 out]
        n226 = property on="SetFormat" class="Bool (strict)"("Val(Sgnl)"=TRUE ("Value (Signaling)")) -> ()  [unwired: 2 in, 2 out]
      }
      event "HMS": Value Change {
        n227 = event-data() -> ("NewVal"=w320:u16)  [unwired: 6 out]
        n228 = property on="SetFormat" class="Bool (strict)"("Val(Sgnl)"=TRUE ("Value (Signaling)")) -> ()  [unwired: 2 in, 2 out]
        n229 = Equal To 0?(x=w320) -> (x = 0?=w321:bool)
        n230 = Select(t=T3."Disabled and Grayed Out" ("Disabled"), s=w321, f=T3."Enabled" ("Disabled")) -> (s? t:f=w318:T3)
        n231 = property on="Digits" class="DigNum (strict)"("DisabledEnum"=w318) -> ()  [unwired: 2 in, 2 out]
      }
      event "DateFormat": Value Change {
        n232 = event-data() -> ("NewVal"=w326:u16)  [unwired: 6 out]
        n233 = case shown="1, 2" w326 {
          tunnel: [T3."Enabled" ("Disabled") T3."Disabled and Grayed Out" ("Disabled")] -> w325
          frame 0, Default {
          }
          frame 1, 2 {
          }
        }
        n234 = property on="SetFormat" class="Bool (strict)"("Val(Sgnl)"=TRUE ("Value (Signaling)")) -> ()  [unwired: 2 in, 2 out]
        n235 = property on="YMD" class="Slide (strict)"("DisabledEnum"=w325) -> ()  [unwired: 2 in, 2 out]
        n236 = property on="YearShow" class="Slide (strict)"("DisabledEnum"=w325) -> ()  [unwired: 2 in, 2 out]
      }
      event "Ignore timestamp information": Value Change {
        n237 = event-data() -> ()  [unwired: 7 out]
        n238 = property on="SetFormat" class="Bool (strict)"("Val(Sgnl)"=TRUE ("Value (Signaling)")) -> ()  [unwired: 2 in, 2 out]
      }
      event "SetFormat": Value Change {
        n239 = event-data() -> ()  [unwired: 7 out]
        n240 = local read "Notation"() -> (w333:i32)
        n241 = case shown="0..3, 5..7, Default" w333 {
          selector: w333 -> [w342 _]
          tunnel: [w351 w390] -> w332
          frame 0..3, 5..7, Default {
            # "%[$][-][+][#][^][0][Width][.Precision || _SignificantDigits][{Unit}][<Embedded information>]Conversion"
            n242 = local read "Exponent in multiples of 3"() -> (w348:bool)
            n243 = local read "Use minimum field width"() -> (w346:bool)
            n244 = local read "Hide trailing zeros"() -> (w349:bool)
            n245 = local read "PrecisionDigits"() -> (w343:u16)
            n246 = local read "PrecisionType"() -> (w344:u16)
            n247 = local read "Field Width"() -> (w345:u16)
            n248 = local read "PadType"() -> (w347:u16)
            n249 = Select(t="#" ("format string"), s=w349, f="" ("format string")) -> (s? t:f=w360:string)
            n250 = Select(t="^" ("format string"), s=w348, f="" ("format string")) -> (s? t:f=w363:string)
            n251 = case shown="True" w346 {
              tunnel: w347 -> [_ w377]
              tunnel: w345 -> [_ w372]
              tunnel: [w369 w376] -> w365
              tunnel: [w369 w370] -> w366
              tunnel: [w369 w375] -> w364
              frame False {
                w369 = ""
              }
              frame True {
                n252 = Not Equal To 0?(x=w372) -> (x != 0?=w373:bool)
                n253 = case shown="2" w377 {
                  tunnel: [w378 "" ("format string") "0" ("format string")] -> w376
                  tunnel: [w378 "-" ("format string") "" ("format string")] -> w375
                  frame 0, Default {
                    w378 = "" ("format string")
                  }
                  frame 1 {
                  }
                  frame 2 {
                  }
                }
                n254 = Number To Decimal String(number=w372) -> (decimal integer string=w371:string)  [unwired: 1 in]
                n255 = Select(t=w371, s=w373, f="") -> (s? t:f=w370:string)
              }
            }
            n256 = Number To Decimal String(number=w343) -> (decimal integer string=w350:string)  [unwired: 1 in]
            n257 = Equal?(x=w344, y=u16 0) -> (x = y?=w357:bool)
            n258 = Index Array(array=string[] ["f", "e", "g", "p", "", "x", "o", "b", "", "T"], index=w342) -> (element=w368:string)
            n259 = Select(t="." ("format string"), s=w357, f="_" ("format string")) -> (s? t:f=w367:string)
            n260 = Concatenate Strings("%" ("string"), w364, w360, w363, w365, w366, w367, w350, w368) -> (w351:string)
          }
          frame 9 {
            n261 = local read "DateFormat"() -> (w385:u16)
            n262 = local read "TimeFormat"() -> (w389:u16)
            n263 = local read "YearShow"() -> (w383:u16)
            n264 = local read "AMFM"() -> (w388:u16)
            n265 = local read "Digits"() -> (w386:u16)
            n266 = local read "HMS"() -> (w387:u16)
            n267 = local read "YMD"() -> (w384:u16)
            n268 = Equal?(x=w385, y=u16 2) -> (x = y?=w405:bool)
            n269 = Equal?(x=w389, y=u16 2) -> (x = y?=w404:bool)
            n270 = case shown="0, Default" w389 {
              tunnel: w388 -> [w464 _ _]
              tunnel: w387 -> [w462 _ _]
              tunnel: w386 -> [w448 w466 _]
              tunnel: [w451 w465 w468] -> w391
              tunnel: w385 -> [_ _ w473]
              frame 0, Default {
                # "Custom Format"
                n271 = Equal To 0?(x=w464) -> (x = 0?=w455:bool)
                n272 = Not Equal To 0?(x=w448) -> (x != 0?=w450:bool)
                n273 = Equal To 0?(x=w462) -> (x = 0?=w459:bool)
                n274 = Format Into String(format string=":%%S%%%du", w448) -> (resulting string=w447:string)  [unwired: 2 in, 1 out]
                n275 = Select(t="%I:%M" ("format string"), s=w455, f="%H:%M" ("format string")) -> (s? t:f=w460:string)
                n276 = Select(t=w447, s=w450, f=":%S" ("format string")) -> (s? t:f=w446:string)
                n277 = Select(t="", s=w459, f=w446) -> (s? t:f=w456:string)
                n278 = Select(t=" %p", s=w455, f="" ("t")) -> (s? t:f=w452:string)
                n279 = Concatenate Strings(w460, w456, w452) -> (w451:string)
              }
              frame 1 {
                # "System Format"
                n280 = Format Into String(format string="%%.%dX", w466) -> (resulting string=w465:string)  [unwired: 2 in, 1 out]
              }
              frame 2 {
                # "No Used"
                n281 = Equal?(x=w473, y=u16 2) -> (x = y?=w471:bool)
                n282 = Select(t="%.3X" ("format string"), s=w471, f="") -> (s? t:f=w468:string)
              }
            }
            n283 = case shown="0, Default" w385 {
              tunnel: w384 -> [w414 _ _]
              tunnel: w383 -> [w413 _ _]
              tunnel: [w411 "%x" ("format string") w440] -> w392
              tunnel: w389 -> [_ _ w441]
              frame 0, Default {
                # "Custom Format"
                n284 = case shown="2" w413 {
                  tunnel: ["" ("format string") "%y" ("format string") "%Y" ("format string")] -> w412
                  frame 0, Default {
                  }
                  frame 1 {
                  }
                  frame 2 {
                  }
                }
                n285 = case shown="2" w414 {
                  tunnel: w412 -> [w419 w426 w434]
                  tunnel: [w423 w430 w438] -> w411
                  frame 0, Default {
                    n286 = Empty String/Path?(string/path=w419) -> (empty?=w422:bool)
                    n287 = Concatenate Strings("/" ("string"), w419) -> (w420:string)
                    n288 = Select(t=w419, s=w422, f=w420) -> (s? t:f=w421:string)
                    n289 = Concatenate Strings("%m/%d" ("format string"), w421) -> (w423:string)
                  }
                  frame 1 {
                    n290 = Empty String/Path?(string/path=w426) -> (empty?=w429:bool)
                    n291 = Concatenate Strings("/" ("string"), w426) -> (w427:string)
                    n292 = Select(t=w426, s=w429, f=w427) -> (s? t:f=w428:string)
                    n293 = Concatenate Strings("%d/%m" ("format string"), w428) -> (w430:string)
                  }
                  frame 2 {
                    n294 = Empty String/Path?(string/path=w434) -> (empty?=w437:bool)
                    n295 = Concatenate Strings(w434, "/" ("string")) -> (w436:string)
                    n296 = Select(t=w434, s=w437, f=w436) -> (s? t:f=w433:string)
                    n297 = Concatenate Strings(w433, "%m/%d" ("format string")) -> (w438:string)
                  }
                }
              }
              frame 1 {
                # "System Format"
              }
              frame 2 {
                # "No Used"
                n298 = Equal?(x=w441, y=u16 2) -> (x = y?=w443:bool)
                n299 = Select(t="%x" ("format string"), s=w443, f="") -> (s? t:f=w440:string)
              }
            }
            n300 = Compound Arithmetic op=AND(w405, w404) -> (w397:bool)
            n301 = Compound Arithmetic op=AND(invert w405, w404) -> (w401:bool)
            n302 = Compound Arithmetic op=AND(w405, invert w404) -> (w402:bool)
            n303 = Compound Arithmetic op=AND(invert w405, invert w404) -> (w406:bool)
            n304 = Compound Arithmetic op=OR(w401, w402) -> (w403:bool)
            n305 = Build Array(w397, w403, w406) -> (w398:bool[])
            n306 = Search 1D Array(1D array=w398, element=TRUE) -> (index of element=w400:i32)  [unwired: 1 in]
            n307 = case shown="2" w400 {
              tunnel: [" " ("format string") "" ("format string") "\n" ("format string")] -> w407
              frame 0, Default {
              }
              frame 1 {
              }
              frame 2 {
              }
            }
            n308 = Concatenate Strings("%<" ("string"), w391, w407, w392, ">T" ("string")) -> (w390:string)
          }
        }
        n309 = property on="FormatAxis" class="Ring (strict)"() -> ("Value"=w331:u16)  [unwired: 2 in, 2 out]
        n310 = case shown="0, Default" w331 {
          tunnel: w330 -> [w335 w338 w341]
          tunnel: w332 -> [w334 w336 w339]
          frame 0, Default {
            n311 = property class="XYGraph"(reference=w335, "XScale.FormatString"=w334) -> ()  [unwired: 1 in, 2 out]
          }
          frame 1 {
            n312 = property class="XYGraph"(reference=w338, "ActYScl"=0 ("Active Y Scale"), "YScale.FormatString"=w336) -> ()  [unwired: 1 in, 2 out]
          }
          frame 2 {
            n313 = property class="XYGraph"(reference=w341, "ActYScl"=1 ("Active Y Scale"), "YScale.FormatString"=w339) -> ()  [unwired: 1 in, 2 out]
          }
        }
      }
      event "LineStyle0", "LineStyle1", "LineStyle2", "LineStyle3", "LineStyle4": Value Change {
        n314 = event-data() -> ("CtlRef"=w480:refnum<vi>)  [unwired: 6 out]
        n315 = property class="Bool (strict)"(reference=w480) -> ("Label.Text"=w478:string)  [unwired: 1 in, 2 out]
        n316 = local read "LineStyle"() -> (w477:string)
        n317 = Equal?(x=w478, y=w477) -> (x = y?=w479:bool)
        n318 = case shown="False" w479 {
          tunnel: w478 -> [w489 w502]
          tunnel: w477 -> [w495 _]
          tunnel: w476 -> [w486 _]
          tunnel: w475 -> [w484 _]
          tunnel: w474 -> [w482 _]
          frame False {
            n319 = control-ref of="This VI"() -> (w496:refnum<vi>)
            n320 = Match Pattern(string=w489, regular expression="LineStyle") -> (after substring=w487:string)  [unwired: 4 out]
            n321 = To Variant(anything=TRUE) -> (Variant=w493:variant)
            n322 = Decimal String To Number(string=w487) -> (number=w483:i32)  [unwired: 3 out]
            n323 = invoke class="VI" method="Ctrl Val.Set"(reference=w496, "Control Name"=w489, "Value"=w493) -> (reference out=w494:refnum<vi>)  [unwired: 2 in, 4 out]
            n324 = To Unsigned Byte Integer(number=w483) -> (unsigned 8bit integer=w481:u8)
            n325 = local write "LineStyle"(w489) -> ()
            n326 = To Variant(anything=FALSE) -> (Variant=w491:variant)
            n327 = property class="XYGraph"(reference=w486, "Plot.Line Style"=w481) -> ()  [unwired: 1 in, 2 out]
            n328 = invoke class="VI" method="Ctrl Val.Set"(reference=w494, "Control Name"=w495, "Value"=w491) -> ()  [unwired: 2 in, 5 out]
            n329 = property on="Items" class="Ring (strict)"() -> ("Value"=w485:u16)  [unwired: 2 in, 2 out]
            n330 = case shown="Default" w482 {
              tunnel: w484 -> [w500 _]
              tunnel: w481 -> [w497 _]
              tunnel: w485 -> [w499 _]
              frame Default {
                n331 = call "CRYSet Plot Settings.vi"("Style"=w497, "sAction"="LineStyle", "Row"=w499, "Legend Refnum"=w500, "Type"=enum16{"Curves", "Values", "Results", "WFM"}."Curves") -> ()  [unwired: 2 in, 5 out]
              }
              frame "ViewReport" {
              }
            }
          }
          frame True {
            n332 = control-ref of="This VI"() -> (w505:refnum<vi>)
            n333 = To Variant(anything=TRUE) -> (Variant=w504:variant)
            n334 = invoke class="VI" method="Ctrl Val.Set"(reference=w505, "Control Name"=w502, "Value"=w504) -> ()  [unwired: 2 in, 5 out]
          }
        }
      }
      event "LineWidth0", "LineWidth1", "LineWidth2", "LineWidth3", "LineWidth4", "LineWidth5": Value Change {
        n335 = event-data() -> ("CtlRef"=w509:refnum<vi>)  [unwired: 6 out]
        n336 = property class="Bool (strict)"(reference=w509) -> ("Label.Text"=w511:string)  [unwired: 1 in, 2 out]
        n337 = local read "LineWidth"() -> (w510:string)
        n338 = Equal?(x=w511, y=w510) -> (x = y?=w512:bool)
        n339 = case shown="False" w512 {
          tunnel: w511 -> [w519 w534]
          tunnel: w510 -> [w527 _]
          tunnel: w508 -> [w517 _]
          tunnel: w507 -> [w515 _]
          tunnel: w506 -> [w514 _]
          frame False {
            n340 = control-ref of="This VI"() -> (w528:refnum<vi>)
            n341 = Match Pattern(string=w519, regular expression="LineWidth") -> (after substring=w520:string)  [unwired: 4 out]
            n342 = To Variant(anything=TRUE) -> (Variant=w525:variant)
            n343 = Decimal String To Number(string=w520) -> (number=w521:i32)  [unwired: 3 out]
            n344 = invoke class="VI" method="Ctrl Val.Set"(reference=w528, "Control Name"=w519, "Value"=w525) -> (reference out=w526:refnum<vi>)  [unwired: 2 in, 4 out]
            n345 = To Unsigned Byte Integer(number=w521) -> (unsigned 8bit integer=w513:u8)
            n346 = local write "LineWidth"(w519) -> ()
            n347 = To Variant(anything=FALSE) -> (Variant=w523:variant)
            n348 = property class="XYGraph"(reference=w517, "Plot.Line Width"=w513) -> ()  [unwired: 1 in, 2 out]
            n349 = invoke class="VI" method="Ctrl Val.Set"(reference=w526, "Control Name"=w527, "Value"=w523) -> ()  [unwired: 2 in, 5 out]
            n350 = property on="Items" class="Ring (strict)"() -> ("Value"=w516:u16)  [unwired: 2 in, 2 out]
            n351 = case shown="Default" w514 {
              tunnel: w515 -> [w532 _]
              tunnel: w513 -> [w529 _]
              tunnel: w516 -> [w531 _]
              frame Default {
                n352 = call "CRYSet Plot Settings.vi"("Style"=w529, "sAction"="LineWidth", "Row"=w531, "Legend Refnum"=w532, "Type"=enum16{"Curves", "Values", "Results", "WFM"}."Curves") -> ()  [unwired: 2 in, 5 out]
              }
              frame "ViewReport" {
              }
            }
          }
          frame True {
            n353 = control-ref of="This VI"() -> (w537:refnum<vi>)
            n354 = To Variant(anything=TRUE) -> (Variant=w536:variant)
            n355 = invoke class="VI" method="Ctrl Val.Set"(reference=w537, "Control Name"=w534, "Value"=w536) -> ()  [unwired: 2 in, 5 out]
          }
        }
      }
      event "PointStyle0", "PointStyle1", "PointStyle2", "PointStyle3", "PointStyle4", "PointStyle5", "PointStyle6", "PointStyle7", "PointStyle8", "PointStyle9", "PointStyle10", "PointStyle11", "PointStyle12", "PointStyle13", "PointStyle14", "PointStyle15", "PointStyle16": Value Change {
        n356 = event-data() -> ("CtlRef"=w541:refnum<vi>)  [unwired: 6 out]
        n357 = property class="Bool (strict)"(reference=w541) -> ("Label.Text"=w543:string)  [unwired: 1 in, 2 out]
        n358 = local read "PointStyle"() -> (w542:string)
        n359 = Equal?(x=w543, y=w542) -> (x = y?=w544:bool)
        n360 = case shown="False" w544 {
          tunnel: w543 -> [w551 w566]
          tunnel: w542 -> [w559 _]
          tunnel: w540 -> [w549 _]
          tunnel: w539 -> [w547 _]
          tunnel: w538 -> [w546 _]
          frame False {
            n361 = control-ref of="This VI"() -> (w560:refnum<vi>)
            n362 = To Variant(anything=TRUE) -> (Variant=w557:variant)
            n363 = Match Pattern(string=w551, regular expression="PointStyle") -> (after substring=w552:string)  [unwired: 4 out]
            n364 = invoke class="VI" method="Ctrl Val.Set"(reference=w560, "Control Name"=w551, "Value"=w557) -> (reference out=w558:refnum<vi>)  [unwired: 2 in, 4 out]
            n365 = Decimal String To Number(string=w552) -> (number=w553:i32)  [unwired: 3 out]
            n366 = local write "PointStyle"(w551) -> ()
            n367 = To Variant(anything=FALSE) -> (Variant=w555:variant)
            n368 = To Unsigned Byte Integer(number=w553) -> (unsigned 8bit integer=w545:u8)
            n369 = invoke class="VI" method="Ctrl Val.Set"(reference=w558, "Control Name"=w559, "Value"=w555) -> ()  [unwired: 2 in, 5 out]
            n370 = property class="XYGraph"(reference=w549, "Plot.Point Style"=w545) -> ()  [unwired: 1 in, 2 out]
            n371 = property on="Items" class="Ring (strict)"() -> ("Value"=w548:u16)  [unwired: 2 in, 2 out]
            n372 = case shown="Default" w546 {
              tunnel: w547 -> [w564 _]
              tunnel: w545 -> [w561 _]
              tunnel: w548 -> [w563 _]
              frame Default {
                n373 = call "CRYSet Plot Settings.vi"("Style"=w561, "sAction"="PointStyle", "Row"=w563, "Legend Refnum"=w564, "Type"=enum16{"Curves", "Values", "Results", "WFM"}."Curves") -> ()  [unwired: 2 in, 5 out]
              }
              frame "ViewReport" {
              }
            }
          }
          frame True {
            n374 = control-ref of="This VI"() -> (w569:refnum<vi>)
            n375 = To Variant(anything=TRUE) -> (Variant=w568:variant)
            n376 = invoke class="VI" method="Ctrl Val.Set"(reference=w569, "Control Name"=w566, "Value"=w568) -> ()  [unwired: 2 in, 5 out]
          }
        }
      }
      event "Interpolation0", "Interpolation1", "Interpolation2", "Interpolation3", "Interpolation4", "Interpolation5": Value Change {
        n377 = event-data() -> ("CtlRef"=w573:refnum<vi>)  [unwired: 6 out]
        n378 = local read "Interpolation"() -> (w574:string)
        n379 = property class="Bool (strict)"(reference=w573) -> ("Label.Text"=w575:string)  [unwired: 1 in, 2 out]
        n380 = Equal?(x=w575, y=w574) -> (x = y?=w576:bool)
        n381 = case shown="False" w576 {
          tunnel: w575 -> [w583 w598]
          tunnel: w574 -> [w591 _]
          tunnel: w572 -> [w581 _]
          tunnel: w571 -> [w579 _]
          tunnel: w570 -> [w578 _]
          frame False {
            n382 = control-ref of="This VI"() -> (w592:refnum<vi>)
            n383 = To Variant(anything=TRUE) -> (Variant=w589:variant)
            n384 = invoke class="VI" method="Ctrl Val.Set"(reference=w592, "Control Name"=w583, "Value"=w589) -> (reference out=w590:refnum<vi>)  [unwired: 2 in, 4 out]
            n385 = Match Pattern(string=w583, regular expression="Interpolation") -> (after substring=w584:string)  [unwired: 4 out]
            n386 = local write "Interpolation"(w583) -> ()
            n387 = To Variant(anything=FALSE) -> (Variant=w587:variant)
            n388 = Decimal String To Number(string=w584) -> (number=w585:i32)  [unwired: 3 out]
            n389 = invoke class="VI" method="Ctrl Val.Set"(reference=w590, "Control Name"=w591, "Value"=w587) -> ()  [unwired: 2 in, 5 out]
            n390 = To Unsigned Byte Integer(number=w585) -> (unsigned 8bit integer=w577:u8)
            n391 = property class="XYGraph"(reference=w581, "Plot.Plot Interpolation"=w577) -> ()  [unwired: 1 in, 2 out]
            n392 = property on="Items" class="Ring (strict)"() -> ("Value"=w580:u16)  [unwired: 2 in, 2 out]
            n393 = case shown="Default" w578 {
              tunnel: w579 -> [w596 _]
              tunnel: w577 -> [w593 _]
              tunnel: w580 -> [w595 _]
              frame Default {
                n394 = call "CRYSet Plot Settings.vi"("Style"=w593, "sAction"="Interpolation", "Row"=w595, "Legend Refnum"=w596, "Type"=enum16{"Curves", "Values", "Results", "WFM"}."Curves") -> ()  [unwired: 2 in, 5 out]
              }
              frame "ViewReport" {
              }
            }
          }
          frame True {
            n395 = control-ref of="This VI"() -> (w601:refnum<vi>)
            n396 = To Variant(anything=TRUE) -> (Variant=w600:variant)
            n397 = invoke class="VI" method="Ctrl Val.Set"(reference=w601, "Control Name"=w598, "Value"=w600) -> ()  [unwired: 2 in, 5 out]
          }
        }
      }
      event "Items": Value Change {
        n398 = event-data() -> ("NewVal"=w603:u16)  [unwired: 6 out]
        n399 = flat-sequence {
          tunnel: w602 -> [w612]
          tunnel: w603 -> [w606]
          tunnel: w604 -> [w608]
          tunnel: [w617] -> w605
          tunnel: w605 -> [w626]
          tunnel: w603 -> [w627]
          tunnel: w602 -> [w625]
          frame #0 {
            n400 = property class="MCListbox"(reference=w608) -> ("ItemSyms"=w611:i32[])  [unwired: 1 in, 2 out]
            n401 = Index Array(array=w611, index=w606) -> (element=w609:i32)
            n402 = Equal?(x=w609, y=38) -> (x = y?=w607:bool)
            n403 = property class="XYGraph"(reference=w612, "Active Plot"=w606, "Plot.Visible?"=w607) -> ()  [unwired: 1 in, 2 out]
            n404 = local write "Show Plot"(w607) -> ()
          }
          frame #1 {
            n405 = control-ref of="This VI"() -> (w617:refnum<vi>)
            n406 = local read "Interpolation"() -> (w613:string)
            n407 = local read "LineWidth"() -> (w615:string)
            n408 = local read "PointStyle"() -> (w614:string)
            n409 = local read "LineStyle"() -> (w616:string)
            n410 = To Variant(anything=FALSE) -> (Variant=w619:variant)
            n411 = invoke class="VI" method="Ctrl Val.Set"(reference=w617, "Control Name"=w616, "Value"=w619) -> ()  [unwired: 2 in, 5 out]
            n412 = invoke class="VI" method="Ctrl Val.Set"(reference=w617, "Control Name"=w615, "Value"=w619) -> ()  [unwired: 2 in, 5 out]
            n413 = invoke class="VI" method="Ctrl Val.Set"(reference=w617, "Control Name"=w614, "Value"=w619) -> ()  [unwired: 2 in, 5 out]
            n414 = invoke class="VI" method="Ctrl Val.Set"(reference=w617, "Control Name"=w613, "Value"=w619) -> ()  [unwired: 2 in, 5 out]
          }
          frame #2 {
            n415 = call "CRYGet Line Infor.vi"("This VI"=w626, "Active Plot Number"=w627, "Graph Type"="OCTAVE", "XY Graph Control Ref"=w625, "Property Set?"=TRUE) -> ("Line"=w620:u32, "Point/Fill"=w621:u32, "Fill to"=w622:i16, "LineStyle"=w631:string, "LineWidth"=w630:string, "PointStyle"=w629:string, "Interpolation"=w628:string)  [unwired: 16 in]
            n416 = local write "Interpolation"(w628) -> ()
            n417 = local write "LineWidth"(w630) -> ()
            n418 = local write "Point/Fill"(w621) -> ()
            n419 = local write "LineStyle"(w631) -> ()
            n420 = local write "PointStyle"(w629) -> ()
            n421 = local write "Fill to"(w622) -> ()
            n422 = local write "Line"(w620) -> ()
          }
        }
      }
      event "Line": Value Change {
        n423 = event-data() -> ("NewVal"=w637:u32)  [unwired: 6 out]
        n424 = property class="XYGraph"(reference=w639, "Plot.Plot Color"=w637) -> ()  [unwired: 1 in, 2 out]
        n425 = property on="Items" class="Ring (strict)"() -> ("Value"=w634:u16)  [unwired: 2 in, 2 out]
        n426 = Bundle By Name(cluster=T4 {"Row"=0, "Column"=0} ("Active Cell:Active Cell"), "Row"=w634, "Column"=1) -> (w635:T4)
        n427 = property class="MCListbox"(reference=w638, "ActiveCell"=w635, "CellBG"=w637) -> ()  [unwired: 1 in, 2 out]
        n428 = case shown="Default" w632 {
          tunnel: w638 -> [w643 _]
          tunnel: w637 -> [w642 _]
          tunnel: w634 -> [w641 _]
          frame Default {
            n429 = call "CRYSet Plot Settings.vi"("sAction"="Color", "Color"=w642, "Row"=w641, "Legend Refnum"=w643, "Type"=enum16{"Curves", "Values", "Results", "WFM"}."Curves") -> ()  [unwired: 2 in, 5 out]
          }
          frame "ViewReport" {
          }
        }
      }
      event "Point/Fill": Value Change {
        n430 = event-data() -> ("NewVal"=w646:u32)  [unwired: 6 out]
        n431 = property class="XYGraph"(reference=w649, "Plot.Fill/Pt. Color"=w646) -> ()  [unwired: 1 in, 2 out]
        n432 = property on="Items" class="Ring (strict)"() -> ("Value"=w648:u16)  [unwired: 2 in, 2 out]
        n433 = case shown="Default" w647 {
          tunnel: w645 -> [w653 _]
          tunnel: w646 -> [w652 _]
          tunnel: w648 -> [w651 _]
          frame Default {
            n434 = call "CRYSet Plot Settings.vi"("sAction"="PointColor", "Color"=w652, "Row"=w651, "Legend Refnum"=w653, "Type"=enum16{"Curves", "Values", "Results", "WFM"}."Curves") -> ()  [unwired: 2 in, 5 out]
          }
          frame "ViewReport" {
          }
        }
      }
      event "Fill to": Value Change {
        n435 = event-data() -> ("NewVal"=w655:i16)  [unwired: 6 out]
        n436 = property class="XYGraph"(reference=w659, "Plot.Fill To"=w655) -> ()  [unwired: 1 in, 2 out]
        n437 = property on="Items" class="Ring (strict)"() -> ("Value"=w658:u16)  [unwired: 2 in, 2 out]
        n438 = case shown="Default" w656 {
          tunnel: w657 -> [w663 _]
          tunnel: w658 -> [w662 _]
          tunnel: w655 -> [w660 _]
          frame Default {
            n439 = call "CRYSet Plot Settings.vi"("Fill To"=w660, "sAction"="FillTo", "Row"=w662, "Legend Refnum"=w663, "Type"=enum16{"Curves", "Values", "Results", "WFM"}."Curves") -> ()  [unwired: 2 in, 5 out]
          }
          frame "ViewReport" {
          }
        }
      }
      event "Show Plot": Value Change {
        w670 = 38
        n440 = event-data() -> ("NewVal"=w675:bool)  [unwired: 6 out]
        n441 = local read "Items"() -> (w667:u16)
        n442 = property class="MCListbox"(reference=w673) -> (reference out=w672:refnum<vi>, "ItemSyms"=w666:i32[])  [unwired: 1 in, 1 out]
        n443 = property class="XYGraph"(reference=w676, "Active Plot"=w667, "Plot.Visible?"=w675) -> ()  [unwired: 1 in, 2 out]
        n444 = Index Array(array=w666, index=w667) -> (element=w674:i32)
        n445 = Equal?(x=w674, y=w670) -> (x = y?=w671:bool)
        n446 = Select(t=37, s=w671, f=w670) -> (s? t:f=w668:i32)
        n447 = Replace Array Subset(array=w666, new element=w668, index=w667) -> (w665:i32[])
        n448 = property class="MCListbox"(reference=w672, "ItemSyms"=w665) -> ()  [unwired: 1 in, 2 out]
      }
      event "Axis": Value Change {
        n449 = event-data() -> ("NewVal"=w699:u16)  [unwired: 6 out]
        n450 = case shown="1" w699 {
          tunnel: w698 -> [w712 w726 w740]
          tunnel: [w711 w725 w739] -> w697
          tunnel: [w710 w724 w738] -> w694
          tunnel: [w709 w723 w737] -> w692
          tunnel: [w708 w722 w736] -> w689
          tunnel: [w707 w721 w735] -> w688
          tunnel: [w706 w720 w734] -> w687
          tunnel: [w705 w719 w733] -> w686
          tunnel: [w704 w718 w732] -> w685
          tunnel: [w703 w717 w731] -> w684
          tunnel: [w702 w716 w730] -> w683
          tunnel: [w701 w715 w729] -> w682
          tunnel: [w700 w713 w727] -> w681
          frame 0, Default {
            n451 = property class="XYGraph"(reference=w712) -> ("XScale.NameLbl.Visible"=w711:bool, "XScale.Style"=w710:u8, "XScale.Mapping Mode"=w709:u8, "XScale.ScaleFit"=w708:u8, "XScale.Maximum"=w707:dbl, "XScale.Minimum"=w706:dbl, "XScale.TickColor"=w705:u32, "XScale.MinorTickColor"=w704:u32, "XScale.Text Color"=w703:u32, "XScale.MajGrdColor"=w702:u32, "XScale.MnrGrdColor"=w701:u32, "XScale.NameLbl.Text"=w700:string)  [unwired: 1 in, 2 out]
          }
          frame 1 {
            n452 = property class="XYGraph"(reference=w726, "ActYScl"=0 ("Active X Scale")) -> ("YScale.NameLbl.Visible"=w725:bool, "YScale.Style"=w724:u8, "YScale.Mapping Mode"=w723:u8, "YScale.ScaleFit"=w722:u8, "YScale.Maximum"=w721:dbl, "YScale.Minimum"=w720:dbl, "YScale.TickColor"=w719:u32, "YScale.MinorTickColor"=w718:u32, "YScale.Text Color"=w717:u32, "YScale.MajGrdColor"=w716:u32, "YScale.MnrGrdColor"=w715:u32, "YScale.NameLbl.Text"=w713:string)  [unwired: 1 in, 2 out]
          }
          frame 2 {
            n453 = property class="XYGraph"(reference=w740, "ActYScl"=1 ("Active X Scale")) -> ("YScale.NameLbl.Visible"=w739:bool, "YScale.Style"=w738:u8, "YScale.Mapping Mode"=w737:u8, "YScale.ScaleFit"=w736:u8, "YScale.Maximum"=w735:dbl, "YScale.Minimum"=w734:dbl, "YScale.TickColor"=w733:u32, "YScale.MinorTickColor"=w732:u32, "YScale.Text Color"=w731:u32, "YScale.MajGrdColor"=w730:u32, "YScale.MnrGrdColor"=w729:u32, "YScale.NameLbl.Text"=w727:string)  [unwired: 1 in, 2 out]
          }
        }
        n454 = Not Equal?(x=w694, y=u8 5 ("X Scale.Scale Fit")) -> (x != y?=w695:bool)
        n455 = Equal?(x=w692, y=u8 1 ("X Scale.Scale Fit")) -> (x = y?=w691:bool)
        n456 = Equal?(x=w689, y=u8 2 ("X Scale.Scale Fit")) -> (x = y?=w677:bool)
        n457 = local write "Show scale label"(w697) -> ()
        n458 = local write "Minor grid"(w682) -> ()
        n459 = local write "Minimum"(w687) -> ()
        n460 = local write "Minor tick"(w685) -> ()
        n461 = local write "Major grid"(w683) -> ()
        n462 = local write "Axis Name"(w681) -> ()
        n463 = local write "Show scale"(w695) -> ()
        n464 = local write "Maximum"(w688) -> ()
        n465 = local write "Major tick"(w686) -> ()
        n466 = local write "Marker text"(w684) -> ()
        n467 = local write "Autoscale"(w677) -> ()
        n468 = local write "Scale Style"(w694) -> ()
        n469 = local write "Log"(w691) -> ()
        n470 = Select(t=u8 2 ("X Scale.Scale Fit"), s=w677, f=u8 0 ("X Scale.Scale Fit")) -> (s? t:f=w678:u8)
        n471 = property on="Maximum" class="DigNum (strict)"("Disabled"=w678) -> ()  [unwired: 2 in, 2 out]
        n472 = property on="Minimum" class="DigNum (strict)"("Disabled"=w678) -> ()  [unwired: 2 in, 2 out]
      }
      event "Axis Name": Value Change {
        n473 = event-data() -> ("NewVal"=w741:string)  [unwired: 6 out]
        n474 = local write "Axis Name"(w741) -> ()
        n475 = local read "Axis"() -> (w743:u16)
        n476 = case shown="2" w743 {
          tunnel: w742 -> [w745 w748 w751]
          tunnel: w741 -> [w744 w746 w749]
          frame 0, Default {
            n477 = property class="XYGraph"(reference=w745, "XScale.NameLbl.Text"=w744) -> ()  [unwired: 1 in, 2 out]
          }
          frame 1 {
            n478 = property class="XYGraph"(reference=w748, "ActYScl"=0 ("Active Y Scale"), "YScale.NameLbl.Text"=w746) -> ()  [unwired: 1 in, 2 out]
          }
          frame 2 {
            n479 = property class="XYGraph"(reference=w751, "ActYScl"=1 ("Active Y Scale"), "YScale.NameLbl.Text"=w749) -> ()  [unwired: 1 in, 2 out]
          }
        }
      }
      event "Show scale label": Value Change {
        n480 = event-data() -> ("NewVal"=w752:bool)  [unwired: 6 out]
        n481 = local read "Axis"() -> (w753:u16)
        n482 = case shown="2" w753 {
          tunnel: w754 -> [w756 w759 w762]
          tunnel: w752 -> [w755 w757 w760]
          frame 0, Default {
            n483 = property class="XYGraph"(reference=w756, "XScale.NameLbl.Visible"=w755) -> ()  [unwired: 1 in, 2 out]
          }
          frame 1 {
            n484 = property class="XYGraph"(reference=w759, "ActYScl"=0 ("Active Y Scale"), "YScale.NameLbl.Visible"=w757) -> ()  [unwired: 1 in, 2 out]
          }
          frame 2 {
            n485 = property class="XYGraph"(reference=w762, "ActYScl"=1 ("Active Y Scale"), "YScale.NameLbl.Visible"=w760) -> ()  [unwired: 1 in, 2 out]
          }
        }
      }
      event "Show scale": Value Change {
        n486 = event-data() -> ("NewVal"=w771:bool)  [unwired: 6 out]
        n487 = local read "Scale Style"() -> (w764:u8)
        n488 = Equal?(x=u8 5 ("X Scale.Scale Fit"), y=w764) -> (x = y?=w766:bool)
        n489 = Select(t=u8 0 ("X Scale.Scale Fit"), s=w766, f=w764) -> (s? t:f=w763:u8)
        n490 = Select(t=w763, s=w771, f=u8 5 ("X Scale.Scale Fit")) -> (s? t:f=w768:u8)
        n491 = local write "Scale Style"(w768) -> ()
        n492 = local read "Axis"() -> (w770:u16)
        n493 = case shown="0, Default" w770 {
          tunnel: w768 -> [w774 w776 w778]
          tunnel: w769 -> [w773 w777 w780]
          frame 0, Default {
            n494 = property class="XYGraph"(reference=w773, "XScale.Style"=w774) -> ()  [unwired: 1 in, 2 out]
          }
          frame 1 {
            n495 = property class="XYGraph"(reference=w777, "ActYScl"=0 ("Active Y Scale"), "YScale.Style"=w776) -> ()  [unwired: 1 in, 2 out]
          }
          frame 2 {
            n496 = property class="XYGraph"(reference=w780, "ActYScl"=1 ("Active Y Scale"), "YScale.Style"=w778) -> ()  [unwired: 1 in, 2 out]
          }
        }
      }
      event "Log": Value Change {
        n497 = event-data() -> ("NewVal"=w784:bool)  [unwired: 6 out]
        n498 = Select(t=u8 1 ("X Scale.Scale Fit"), s=w784, f=u8 0 ("X Scale.Scale Fit")) -> (s? t:f=w782:u8)
        n499 = local read "Axis"() -> (w783:u16)
        n500 = case shown="2" w783 {
          tunnel: w782 -> [w788 w790 w792]
          tunnel: w781 -> [w787 w791 w794]
          frame 0, Default {
            n501 = property class="XYGraph"(reference=w787, "XScale.Mapping Mode"=w788) -> ()  [unwired: 1 in, 2 out]
          }
          frame 1 {
            n502 = property class="XYGraph"(reference=w791, "ActYScl"=0 ("Active Y Scale"), "YScale.Mapping Mode"=w790) -> ()  [unwired: 1 in, 2 out]
          }
          frame 2 {
            n503 = property class="XYGraph"(reference=w794, "ActYScl"=1 ("Active Y Scale"), "YScale.Mapping Mode"=w792) -> ()  [unwired: 1 in, 2 out]
          }
        }
      }
      event "GridStyle": Value Change {
        n504 = event-data() -> ("NewVal"=w796:u16)  [unwired: 6 out]
        n505 = local read "Axis"() -> (w797:u16)
        n506 = case shown="0, Default" w797 {
          tunnel: w796 -> [w799 w801 w803]
          tunnel: w795 -> [w798 w802 w805]
          frame 0, Default {
            n507 = property class="XYGraph"(reference=w798, "XScale.Style"=w799) -> ()  [unwired: 1 in, 2 out]
          }
          frame 1 {
            n508 = property class="XYGraph"(reference=w802, "ActYScl"=0 ("Active Y Scale"), "YScale.Style"=w801) -> ()  [unwired: 1 in, 2 out]
          }
          frame 2 {
            n509 = property class="XYGraph"(reference=w805, "ActYScl"=1 ("Active Y Scale"), "YScale.Style"=w803) -> ()  [unwired: 1 in, 2 out]
          }
        }
      }
      event "Major tick": Value Change {
        n510 = event-data() -> ("NewVal"=w806:u32)  [unwired: 6 out]
        n511 = local read "Axis"() -> (w808:u16)
        n512 = case shown="0, Default" w808 {
          tunnel: w807 -> [w810 w813 w816]
          tunnel: w806 -> [w809 w811 w814]
          frame 0, Default {
            n513 = property class="XYGraph"(reference=w810, "XScale.TickColor"=w809) -> ()  [unwired: 1 in, 2 out]
          }
          frame 1 {
            n514 = property class="XYGraph"(reference=w813, "ActYScl"=0 ("Active Y Scale"), "YScale.TickColor"=w811) -> ()  [unwired: 1 in, 2 out]
          }
          frame 2 {
            n515 = property class="XYGraph"(reference=w816, "ActYScl"=1 ("Active Y Scale"), "YScale.TickColor"=w814) -> ()  [unwired: 1 in, 2 out]
          }
        }
      }
      event "Minor tick": Value Change {
        n516 = event-data() -> ("NewVal"=w817:u32)  [unwired: 6 out]
        n517 = local read "Axis"() -> (w819:u16)
        n518 = case shown="0, Default" w819 {
          tunnel: w817 -> [w821 w823 w825]
          tunnel: w818 -> [w820 w824 w827]
          frame 0, Default {
            n519 = property class="XYGraph"(reference=w820, "XScale.MinorTickColor"=w821) -> ()  [unwired: 1 in, 2 out]
          }
          frame 1 {
            n520 = property class="XYGraph"(reference=w824, "ActYScl"=0 ("Active Y Scale"), "YScale.MinorTickColor"=w823) -> ()  [unwired: 1 in, 2 out]
          }
          frame 2 {
            n521 = property class="XYGraph"(reference=w827, "ActYScl"=1 ("Active Y Scale"), "YScale.MinorTickColor"=w825) -> ()  [unwired: 1 in, 2 out]
          }
        }
      }
      event "Marker text": Value Change {
        n522 = event-data() -> ("NewVal"=w828:u32)  [unwired: 6 out]
        n523 = local read "Axis"() -> (w830:u16)
        n524 = case shown="0, Default" w830 {
          tunnel: w828 -> [w832 w834 w836]
          tunnel: w829 -> [w831 w835 w838]
          frame 0, Default {
            n525 = property class="XYGraph"(reference=w831, "XScale.Text Color"=w832) -> ()  [unwired: 1 in, 2 out]
          }
          frame 1 {
            n526 = property class="XYGraph"(reference=w835, "ActYScl"=0 ("Active Y Scale"), "YScale.Text Color"=w834) -> ()  [unwired: 1 in, 2 out]
          }
          frame 2 {
            n527 = property class="XYGraph"(reference=w838, "ActYScl"=1 ("Active Y Scale"), "YScale.Text Color"=w836) -> ()  [unwired: 1 in, 2 out]
          }
        }
      }
      event "Major grid": Value Change {
        n528 = event-data() -> ("NewVal"=w840:u32)  [unwired: 6 out]
        n529 = local read "Axis"() -> (w841:u16)
        n530 = case shown="0, Default" w841 {
          tunnel: w840 -> [w843 w845 w847]
          tunnel: w839 -> [w842 w846 w849]
          frame 0, Default {
            n531 = property class="XYGraph"(reference=w842, "XScale.MajGrdColor"=w843) -> ()  [unwired: 1 in, 2 out]
          }
          frame 1 {
            n532 = property class="XYGraph"(reference=w846, "ActYScl"=0 ("Active Y Scale"), "YScale.MajGrdColor"=w845) -> ()  [unwired: 1 in, 2 out]
          }
          frame 2 {
            n533 = property class="XYGraph"(reference=w849, "ActYScl"=1 ("Active Y Scale"), "YScale.MajGrdColor"=w847) -> ()  [unwired: 1 in, 2 out]
          }
        }
      }
      event "Minor grid": Value Change {
        n534 = event-data() -> ("NewVal"=w850:u32)  [unwired: 6 out]
        n535 = local read "Axis"() -> (w852:u16)
        n536 = case shown="0, Default" w852 {
          tunnel: w850 -> [w854 w856 w858]
          tunnel: w851 -> [w853 w857 w860]
          frame 0, Default {
            n537 = property class="XYGraph"(reference=w853, "XScale.MnrGrdColor"=w854) -> ()  [unwired: 1 in, 2 out]
          }
          frame 1 {
            n538 = property class="XYGraph"(reference=w857, "ActYScl"=0 ("Active Y Scale"), "YScale.MnrGrdColor"=w856) -> ()  [unwired: 1 in, 2 out]
          }
          frame 2 {
            n539 = property class="XYGraph"(reference=w860, "ActYScl"=1 ("Active Y Scale"), "YScale.MnrGrdColor"=w858) -> ()  [unwired: 1 in, 2 out]
          }
        }
      }
      event "Autoscale": Value Change {
        n540 = event-data() -> ("NewVal"=w861:bool)  [unwired: 6 out]
        n541 = local read "Axis"() -> (w872:u16)
        n542 = Select(t=u8 2 ("X Scale.Scale Fit"), s=w861, f=u8 0 ("X Scale.Scale Fit")) -> (s? t:f=w876:u8)
        n543 = local read "Maximum"() -> (w871:dbl)
        n544 = local read "Minimum"() -> (w870:dbl)
        n545 = Select(t=u8 2 ("X Scale.Scale Fit"), s=w861, f=u8 0 ("X Scale.Scale Fit")) -> (s? t:f=w875:u8)
        n546 = case shown="False" w861 {
          tunnel: w872 -> [w882 _]
          tunnel: w871 -> [w881 _]
          tunnel: w870 -> [w880 _]
          tunnel: w869 -> [w879 _]
          frame False {
            n547 = case shown="0, Default" w882 {
              tunnel: w879 -> [w885 w889 w893]
              tunnel: w881 -> [w884 w887 w891]
              tunnel: w880 -> [w883 w886 w890]
              frame 0, Default {
                n548 = property class="XYGraph"(reference=w885, "XScale.Maximum"=w884, "XScale.Minimum"=w883) -> ()  [unwired: 1 in, 2 out]
              }
              frame 1 {
                n549 = property class="XYGraph"(reference=w889, "ActYScl"=0 ("Active Y Scale"), "YScale.Maximum"=w887, "YScale.Minimum"=w886) -> ()  [unwired: 1 in, 2 out]
              }
              frame 2 {
                n550 = property class="XYGraph"(reference=w893, "ActYScl"=1 ("Active Y Scale"), "YScale.Maximum"=w891, "YScale.Minimum"=w890) -> ()  [unwired: 1 in, 2 out]
              }
            }
          }
          frame True {
          }
        }
        n551 = case shown="2" w872 {
          tunnel: w876 -> [w895 w899 w902]
          tunnel: w869 -> [w896 w900 w904]
          tunnel: ["ScaleFitX" ("Label Name") "ScaleFitY" ("Label Name") "ScaleFitY 2" ("Label Name")] -> w862
          frame 0, Default {
            n552 = property class="XYGraph"(reference=w896, "XScale.ScaleFit"=w895) -> ()  [unwired: 1 in, 2 out]
          }
          frame 1 {
            n553 = property class="XYGraph"(reference=w900, "ActYScl"=0 ("Active Y Scale"), "YScale.ScaleFit"=w899) -> ()  [unwired: 1 in, 2 out]
          }
          frame 2 {
            n554 = property class="XYGraph"(reference=w904, "ActYScl"=1 ("Active Y Scale"), "YScale.ScaleFit"=w902) -> ()  [unwired: 1 in, 2 out]
          }
        }
        n555 = property on="Maximum" class="DigNum (strict)"("Disabled"=w875) -> ()  [unwired: 2 in, 2 out]
        n556 = property on="Minimum" class="DigNum (strict)"("Disabled"=w875) -> ()  [unwired: 2 in, 2 out]
        n557 = call "CRYGet Boolean Reference.vi"("Label Name"=w862, "VI Refnum"=w863) -> ("Boolean Ref"=w868:refnum<vi>, "VI Refnum Out"=w867:refnum<vi>)  [unwired: 7 in, 1 out]
        n558 = property class="Bool"(reference=w868, "Value"=w861) -> (error out=w864:errorcluster)  [unwired: 1 in, 1 out]
        n559 = call "CRYGet Boolean Reference.vi"("Label Name"="ToolbarUpdate", "VI Refnum"=w867) -> ("Boolean Ref"=w865:refnum<vi>)  [unwired: 7 in, 2 out]
        n560 = property class="Bool"(reference=w865, error in=w864, "Val(Sgnl)"=w861) -> ()  [unwired: 2 out]
      }
      event "Maximum": Value Change {
        n561 = event-data() -> ("NewVal"=w905:dbl)  [unwired: 6 out]
        n562 = local read "Axis"() -> (w907:u16)
        n563 = case shown="0, Default" w907 {
          tunnel: w905 -> [w909 w911 w913]
          tunnel: w906 -> [w908 w912 w915]
          frame 0, Default {
            n564 = property class="XYGraph"(reference=w908, "XScale.Maximum"=w909) -> ()  [unwired: 1 in, 2 out]
          }
          frame 1 {
            n565 = property class="XYGraph"(reference=w912, "ActYScl"=0 ("Active Y Scale"), "YScale.Maximum"=w911) -> ()  [unwired: 1 in, 2 out]
          }
          frame 2 {
            n566 = property class="XYGraph"(reference=w915, "ActYScl"=1 ("Active Y Scale"), "YScale.Maximum"=w913) -> ()  [unwired: 1 in, 2 out]
          }
        }
        n567 = local write "Maximum"(w905) -> ()
      }
      event "Minimum": Value Change {
        n568 = event-data() -> ("NewVal"=w916:dbl)  [unwired: 6 out]
        n569 = local read "Axis"() -> (w918:u16)
        n570 = case shown="0, Default" w918 {
          tunnel: w916 -> [w920 w922 w924]
          tunnel: w917 -> [w919 w923 w926]
          frame 0, Default {
            n571 = property class="XYGraph"(reference=w919, "XScale.Minimum"=w920) -> ()  [unwired: 1 in, 2 out]
          }
          frame 1 {
            n572 = property class="XYGraph"(reference=w923, "ActYScl"=0 ("Active Y Scale"), "YScale.Minimum"=w922) -> ()  [unwired: 1 in, 2 out]
          }
          frame 2 {
            n573 = property class="XYGraph"(reference=w926, "ActYScl"=1 ("Active Y Scale"), "YScale.Minimum"=w924) -> ()  [unwired: 1 in, 2 out]
          }
        }
        n574 = local write "Minimum"(w916) -> ()
      }
      event "Show Cursors": Value Change {
        n575 = event-data() -> ("NewVal"=w927:bool)  [unwired: 6 out]
        n576 = local write "Show Cursors"(w927) -> ()
        n577 = Select(t=0, s=w927, f=2) -> (s? t:f=w931:i32)
        n578 = call "CRYGet Boolean Reference.vi"("Label Name"="CursorShow", "VI Refnum"=w930) -> ("Boolean Ref"=w929:refnum<vi>)  [unwired: 7 in, 2 out]
        n579 = property on="Cursor Tab" class="TabCtl (strict)"("DisabledEnum"=w931) -> ()  [unwired: 2 in, 2 out]
        n580 = property class="Bool"(reference=w929, "Val(Sgnl)"=w927) -> ()  [unwired: 1 in, 2 out]
      }
      event "Cursor Items": Value Change {
        n581 = event-data() -> ("NewVal"=w935:u16)  [unwired: 6 out]
        n582 = flat-sequence {
          tunnel: [w942] -> w936
          tunnel: w936 -> [w946]
          tunnel: w935 -> [w944]
          tunnel: w934 -> [w945]
          frame #0 {
            n583 = local read "CursorLineWidth"() -> (w940:string)
            n584 = local read "CursorPointStyle"() -> (w939:string)
            n585 = local read "CursorLineStyle"() -> (w941:string)
            n586 = control-ref of="This VI"() -> (w942:refnum<vi>)
            n587 = local read "CursorStyle"() -> (w938:string)
            n588 = To Variant(anything=FALSE) -> (Variant=w943:variant)
            n589 = invoke class="VI" method="Ctrl Val.Set"(reference=w942, "Control Name"=w941, "Value"=w943) -> ()  [unwired: 2 in, 5 out]
            n590 = invoke class="VI" method="Ctrl Val.Set"(reference=w942, "Control Name"=w940, "Value"=w943) -> ()  [unwired: 2 in, 5 out]
            n591 = invoke class="VI" method="Ctrl Val.Set"(reference=w942, "Control Name"=w939, "Value"=w943) -> ()  [unwired: 2 in, 5 out]
            n592 = invoke class="VI" method="Ctrl Val.Set"(reference=w942, "Control Name"=w938, "Value"=w943) -> ()  [unwired: 2 in, 5 out]
          }
          frame #1 {
            n593 = call "CRYSet Cursor Infor.vi"("This VI"=w946, "Active Cursor"=w944, "Graph Type"="OCTAVE", "XY Graph Ref"=w945, "Property Set?"=TRUE) -> ("Cursor Color"=w947:u32, "CursorLineStyle"=w950:string, "CursorLineWidth"=w951:string, "CursorPointStyle"=w952:string, "CursorStyle"=w953:string)  [unwired: 17 in, 1 out]
            n594 = local write "CursorLineWidth"(w951) -> ()
            n595 = local write "Cursor color"(w947) -> ()
            n596 = local write "CursorLineStyle"(w950) -> ()
            n597 = local write "CursorPointStyle"(w952) -> ()
            n598 = local write "CursorStyle"(w953) -> ()
          }
        }
      }
      event "CursorLineStyle0", "CursorLineStyle1", "CursorLineStyle2", "CursorLineStyle3", "CursorLineStyle4": Value Change {
        n599 = event-data() -> ("CtlRef"=w955:refnum<vi>)  [unwired: 6 out]
        n600 = local read "CursorLineStyle"() -> (w956:string)
        n601 = property class="Bool (strict)"(reference=w955) -> ("Label.Text"=w957:string)  [unwired: 1 in, 2 out]
        n602 = Equal?(x=w957, y=w956) -> (x = y?=w958:bool)
        n603 = case shown="False" w958 {
          tunnel: w957 -> [w963 w971]
          tunnel: w956 -> [w969 _]
          tunnel: w954 -> [w959 _]
          frame False {
            n604 = control-ref of="This VI"() -> (w970:refnum<vi>)
            n605 = Match Pattern(string=w963, regular expression="CursorLineStyle") -> (after substring=w961:string)  [unwired: 4 out]
            n606 = To Variant(anything=TRUE) -> (Variant=w967:variant)
            n607 = Decimal String To Number(string=w961) -> (number=w960:i32)  [unwired: 3 out]
            n608 = invoke class="VI" method="Ctrl Val.Set"(reference=w970, "Control Name"=w963, "Value"=w967) -> (reference out=w968:refnum<vi>)  [unwired: 2 in, 4 out]
            n609 = local write "CursorLineStyle"(w963) -> ()
            n610 = property class="XYGraph"(reference=w959, "Cursor.LineStyle"=w960) -> ()  [unwired: 1 in, 2 out]
            n611 = To Variant(anything=FALSE) -> (Variant=w965:variant)
            n612 = invoke class="VI" method="Ctrl Val.Set"(reference=w968, "Control Name"=w969, "Value"=w965) -> ()  [unwired: 2 in, 5 out]
          }
          frame True {
            n613 = control-ref of="This VI"() -> (w974:refnum<vi>)
            n614 = To Variant(anything=TRUE) -> (Variant=w973:variant)
            n615 = invoke class="VI" method="Ctrl Val.Set"(reference=w974, "Control Name"=w971, "Value"=w973) -> ()  [unwired: 2 in, 5 out]
          }
        }
      }
      event "CursorLineWidth0", "CursorLineWidth1", "CursorLineWidth2", "CursorLineWidth3", "CursorLineWidth4", "CursorLineWidth5": Value Change {
        n616 = event-data() -> ("CtlRef"=w976:refnum<vi>)  [unwired: 6 out]
        n617 = local read "CursorLineWidth"() -> (w977:string)
        n618 = property class="Bool (strict)"(reference=w976) -> ("Label.Text"=w978:string)  [unwired: 1 in, 2 out]
        n619 = Equal?(x=w978, y=w977) -> (x = y?=w979:bool)
        n620 = case shown="False" w979 {
          tunnel: w978 -> [w982 w992]
          tunnel: w977 -> [w990 _]
          tunnel: w975 -> [w980 _]
          frame False {
            n621 = control-ref of="This VI"() -> (w991:refnum<vi>)
            n622 = Match Pattern(string=w982, regular expression="CursorLineWidth") -> (after substring=w983:string)  [unwired: 4 out]
            n623 = To Variant(anything=TRUE) -> (Variant=w988:variant)
            n624 = Decimal String To Number(string=w983) -> (number=w984:i32)  [unwired: 3 out]
            n625 = invoke class="VI" method="Ctrl Val.Set"(reference=w991, "Control Name"=w982, "Value"=w988) -> (reference out=w989:refnum<vi>)  [unwired: 2 in, 4 out]
            n626 = local write "CursorLineWidth"(w982) -> ()
            n627 = property class="XYGraph"(reference=w980, "Cursor.LineWidth"=w984) -> ()  [unwired: 1 in, 2 out]
            n628 = To Variant(anything=FALSE) -> (Variant=w986:variant)
            n629 = invoke class="VI" method="Ctrl Val.Set"(reference=w989, "Control Name"=w990, "Value"=w986) -> ()  [unwired: 2 in, 5 out]
          }
          frame True {
            n630 = control-ref of="This VI"() -> (w995:refnum<vi>)
            n631 = To Variant(anything=TRUE) -> (Variant=w994:variant)
            n632 = invoke class="VI" method="Ctrl Val.Set"(reference=w995, "Control Name"=w992, "Value"=w994) -> ()  [unwired: 2 in, 5 out]
          }
        }
      }
      event "CursorPointStyle0", "CursorPointStyle1", "CursorPointStyle2", "CursorPointStyle3", "CursorPointStyle4", "CursorPointStyle5", "CursorPointStyle6", "CursorPointStyle7", "CursorPointStyle8", "CursorPointStyle9", "CursorPointStyle10", "CursorPointStyle11", "CursorPointStyle12", "CursorPointStyle13", "CursorPointStyle14", "CursorPointStyle15", "CursorPointStyle16": Value Change {
        n633 = event-data() -> ("CtlRef"=w997:refnum<vi>)  [unwired: 6 out]
        n634 = local read "CursorPointStyle"() -> (w998:string)
        n635 = property class="Bool (strict)"(reference=w997) -> ("Label.Text"=w999:string)  [unwired: 1 in, 2 out]
        n636 = Equal?(x=w999, y=w998) -> (x = y?=w1000:bool)
        n637 = case shown="False" w1000 {
          tunnel: w999 -> [w1003 w1013]
          tunnel: w998 -> [w1011 _]
          tunnel: w996 -> [w1001 _]
          frame False {
            n638 = control-ref of="This VI"() -> (w1012:refnum<vi>)
            n639 = To Variant(anything=TRUE) -> (Variant=w1009:variant)
            n640 = Match Pattern(string=w1003, regular expression="CursorPointStyle") -> (after substring=w1004:string)  [unwired: 4 out]
            n641 = invoke class="VI" method="Ctrl Val.Set"(reference=w1012, "Control Name"=w1003, "Value"=w1009) -> (reference out=w1010:refnum<vi>)  [unwired: 2 in, 4 out]
            n642 = local write "CursorPointStyle"(w1003) -> ()
            n643 = Decimal String To Number(string=w1004) -> (number=w1005:i32)  [unwired: 3 out]
            n644 = property class="XYGraph"(reference=w1001, "Cursor.Cursor Point Style"=w1005) -> ()  [unwired: 1 in, 2 out]
            n645 = To Variant(anything=FALSE) -> (Variant=w1007:variant)
            n646 = invoke class="VI" method="Ctrl Val.Set"(reference=w1010, "Control Name"=w1011, "Value"=w1007) -> ()  [unwired: 2 in, 5 out]
          }
          frame True {
            n647 = control-ref of="This VI"() -> (w1016:refnum<vi>)
            n648 = To Variant(anything=TRUE) -> (Variant=w1015:variant)
            n649 = invoke class="VI" method="Ctrl Val.Set"(reference=w1016, "Control Name"=w1013, "Value"=w1015) -> ()  [unwired: 2 in, 5 out]
          }
        }
      }
      event "CursorStyle0", "CursorStyle1", "CursorStyle2", "CursorStyle3", "CursorStyle6", "CursorStyle7", "CursorStyle5", "CursorStyle4", "CursorStyle8": Value Change {
        n650 = event-data() -> ("CtlRef"=w1018:refnum<vi>)  [unwired: 6 out]
        n651 = local read "CursorStyle"() -> (w1019:string)
        n652 = property class="Bool (strict)"(reference=w1018) -> ("Label.Text"=w1020:string)  [unwired: 1 in, 2 out]
        n653 = Equal?(x=w1020, y=w1019) -> (x = y?=w1021:bool)
        n654 = case shown="False" w1021 {
          tunnel: w1020 -> [w1024 w1034]
          tunnel: w1019 -> [w1032 _]
          tunnel: w1017 -> [w1022 _]
          frame False {
            n655 = control-ref of="This VI"() -> (w1033:refnum<vi>)
            n656 = To Variant(anything=TRUE) -> (Variant=w1030:variant)
            n657 = Match Pattern(string=w1024, regular expression="CursorStyle") -> (after substring=w1025:string)  [unwired: 4 out]
            n658 = invoke class="VI" method="Ctrl Val.Set"(reference=w1033, "Control Name"=w1024, "Value"=w1030) -> (reference out=w1031:refnum<vi>)  [unwired: 2 in, 4 out]
            n659 = Decimal String To Number(string=w1025) -> (number=w1026:i32)  [unwired: 3 out]
            n660 = local write "CursorStyle"(w1024) -> ()
            n661 = property class="XYGraph"(reference=w1022, "Cursor.Cursor Style"=w1026) -> ()  [unwired: 1 in, 2 out]
            n662 = To Variant(anything=FALSE) -> (Variant=w1028:variant)
            n663 = invoke class="VI" method="Ctrl Val.Set"(reference=w1031, "Control Name"=w1032, "Value"=w1028) -> ()  [unwired: 2 in, 5 out]
          }
          frame True {
            n664 = control-ref of="This VI"() -> (w1037:refnum<vi>)
            n665 = To Variant(anything=TRUE) -> (Variant=w1036:variant)
            n666 = invoke class="VI" method="Ctrl Val.Set"(reference=w1037, "Control Name"=w1034, "Value"=w1036) -> ()  [unwired: 2 in, 5 out]
          }
        }
      }
      event "Cursor color": Value Change {
        n667 = event-data() -> ("NewVal"=w1045:u32)  [unwired: 6 out]
        n668 = local read "Cursor Items"() -> (w1044:u16)
        n669 = property class="XYGraph"(reference=w1042) -> (reference out=w1041:refnum<vi>, "Active Cursor"=w1039:u32)  [unwired: 1 in, 1 out]
        n670 = local write "Cursor color"(w1045) -> ()
        n671 = property class="XYGraph"(reference=w1041, "Active Cursor"=w1044, "Cursor.Cursor Color"=w1045) -> (reference out=w1040:refnum<vi>)  [unwired: 1 in, 1 out]
        n672 = property class="XYGraph"(reference=w1040, "Active Cursor"=w1039) -> (reference out=w1038:refnum<vi>)  [unwired: 1 in, 1 out]
        n673 = flat-sequence {
          tunnel: w1043 -> [w1046]
          tunnel: w1038 -> [_]
          frame #0 {
            n674 = call "CRYGet Boolean Reference.vi"("Label Name"="CursorColor" ("Control Name"), "VI Refnum"=w1046) -> ("Boolean Ref"=w1048:refnum<vi>)  [unwired: 7 in, 2 out]
            n675 = property class="Bool"(reference=w1048, "Val(Sgnl)"=TRUE ("Visible")) -> ()  [unwired: 1 in, 2 out]
          }
        }
      }
      event "Linked to plot:": Value Change {
        n676 = event-data() -> ("NewVal"=w1050:u16)  [unwired: 6 out]
        n677 = local write "Linked to plot:"(w1050) -> ()
        n678 = local read "Cursor Items"() -> (w1052:u16)
        n679 = property class="XYGraph"(reference=w1051, "Active Cursor"=w1052, "Cursor.Cursor Plot"=w1050) -> ()  [unwired: 1 in, 2 out]
      }
      event "Link Cursors": Value Change {
        n680 = event-data() -> ("NewVal"=w1053:bool)  [unwired: 6 out]
        n681 = local write "Link Cursors"(w1053) -> ()
      }
    }
  }
